vi "MainPr(Calculation)-40.vi"() -> ()   [LabVIEW 2013]
doc: "Main Program for Tracking\nThis VI Represents Front Panel and Control Buttons for Perform Tracking\nPlease, optimize the front panel for your own monitor resolution and needs"
uses:
  <vilib>/vision/Avi.llb/IMAQ AVI2 Refnum.ctl
  <vilib>/vision/NI_Vision_Development_Module.lvlib
panel:
  out "error out":errorcluster
  in  "STOP Program":bool
  in  "Front Panel":T1(tab)
  in  "FrameCtl":u32 max=499
  out "1st Movie (Comparison)":T2(plugin-control)
  out "1st Movie":T2(plugin-control)
  in  "Gamma":sgl format="%.2f"
  in  "Operator G Correction":T3(ring)
  in  "Parameter LoG":sgl format="%.2f"
  in  "Operator LoG":T3(ring)
  in  "1/2 Channels":bool
  in  "Sigma":dbl min=0.1
  in  "FrameCtl2":u32 max=499
  in  "Gray or Binarized?":bool
  out "1st Movie Original":T2(plugin-control)
  out "1st Movie Processed":T2(plugin-control)
  in  "Index for thresholding":i8 min=-9
  in  "Keep Nega-\ntive Values?":bool
  out "Detection Progress":u8(slide) scale=0.0..100.0
  in  "# of Frame":u32 max=499
  in  "Save pics (ex)":bool
  in  "Find ALL objects":bool
  out "Results on 1st Movie":T2(plugin-control)
  out "1st Filtering":T2(plugin-control)
  in  "Try my filters!":bool
  in  "# Erosion":i32=2
  in  "Connectivity":bool=TRUE
  in  "Min  Diam":dbl
  in  "Max  Diam":dbl min=12.0
  in  "Filter Tracks":bool
  out "Tracking progress":u8(slide) scale=0.0..100.0
  in  "Save pictures":bool
  in  "Save movies":bool
  in  "Frame":u32 max=499
  in  "Delete Tracs":bool
  out "1st Filtered":T2(plugin-control)
  in  "dR max":dbl min=1.0
  out "1st Filtering (NN)":T2(plugin-control)
  in  "dR min":dbl min=0.0 max=10.0
  out "Raw #":i32
  out "Saved #":i32
  in  "Tracking Procedure":bool
  in  "Min TRK L":i32 min=2 max=498 step=1
  in  "Closing gaps":i32 min=1 max=498 step=1
  in  "% linearity":i32 min=1 max=100 step=1
  in  "Max angle":dbl min=0.0 max=89.0 step=1.0
  in  "FPS":u32
  in  "FPS Gr":u32
  in  "Save videos \nbelow as *avi":bool
  in  "Save pics below":bool
  in  "Testing Frame":u32 max=17
  out "After Resolving Correspondence Problem":T2(plugin-control)
  out "Connected and Grouped Tracks":T2(plugin-control)
  in  "Tracks group":i32 min=0 max=394
  in  "Save Tracks in Columns (x,y,dx,dy)":bool
  in  "Save Duration of Tracks":bool
  in  "Save Mean Velocities":bool
  out "Duration of Tracks":T4(graph)
  out "Mean Instant Velocities for Each Track":T4(graph)
  in  "Show Distributions":bool
  out "All Path Vels":T4(graph)
  out "All Instant Vels":T4(graph)
  out "mean Instant Vel":dbl format="%#_1f"
  out "StD Instant":dbl format="%#_1g"
  out "mean Path Vel":dbl format="%.1f"
  out "StD Path":dbl format="%.1f"
  in  "Bins":i32=10
  in  "Save All Instant Vels":bool
  in  "Save Path Velocities":bool
  # "Two channels"
  # "*Planning develop-\nment switcher (old)"
  # "One channel"
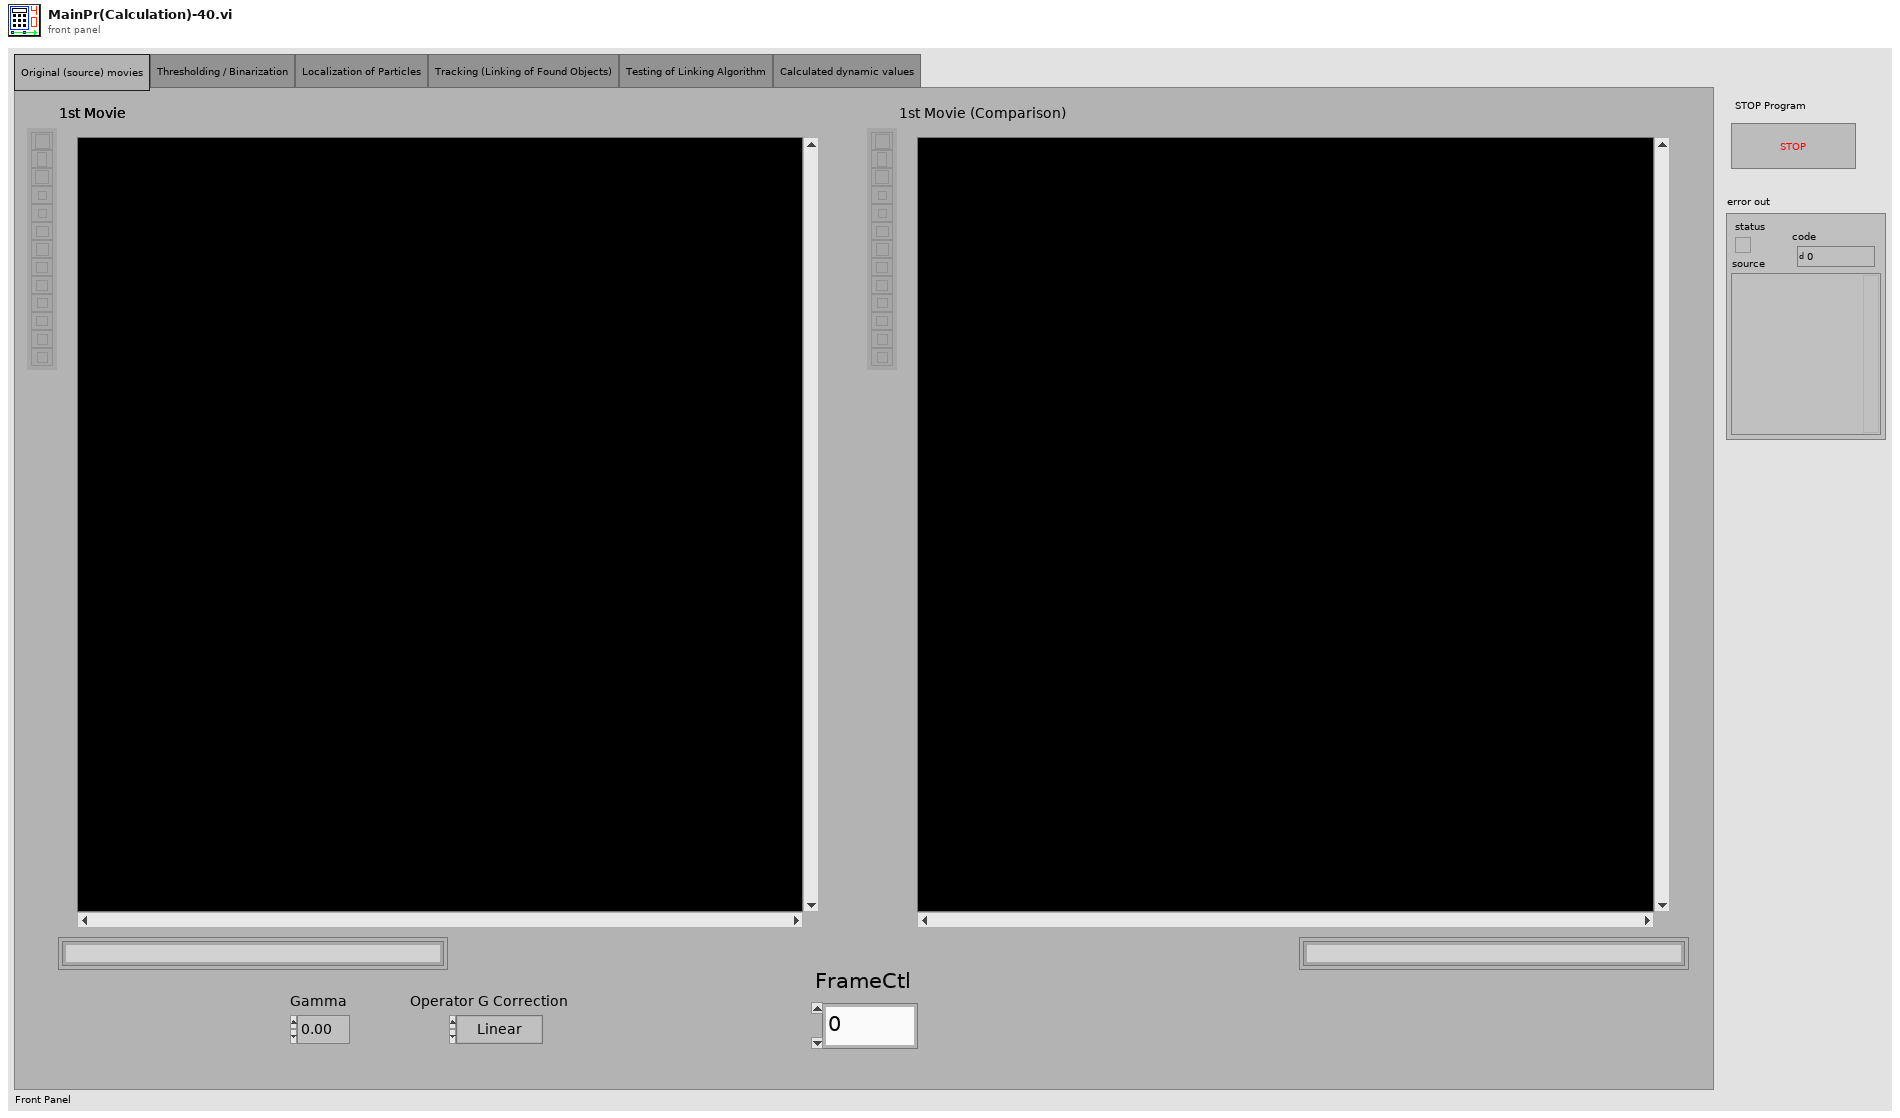
[diagram p1: front panel]
types:
  T1 = enum32{"Original (source) movies", "Thresholding / Binarization", "Localization of Particles", "Tracking (Linking of Found Objects)", "Testing of Linking Algorithm", "Calculated dynamic values"}
  T2 = typedef "IMAQ Image.ctl" = refnum<image>
  T3 = enum32{"Linear", "Log", "Exp", "Square", "Square root", "Power X", "Power 1/X"}
  T4 = cluster{"X Values":dbl[], "Histogram: h(x)":i32[]}
  T5 = typedef "IMAQ AVI2 Refnum.ctl" = refnum<k20>
  T6 = typedef "Image Type" = u32
  T7 = typedef "Particle Parameters" = i32
  T8 = cluster{"[IN] AVI Refnum":T5, "[IN] Image Type":T6, "[IN] Particle Filter Setups":cluster{"Erosion":i32, "Connectivity ":bool, "Type of particle filter":cluster{"Measurement Parameter":T7, "Min  Diam":dbl, "Max  Diam":dbl, "Range":bool, "Range":bool}[]}, "[IN] # Channel":u8, "[IN] Keep Nega-\ntive Values?":bool, "[IN] Image Filtering Settings":cluster{"Gamma Origin":sgl, "Operator Origin":enum32{"Linear", "Log", "Exp", "Square", "Square root", "Power X", "Power 1/X"}, "Gamma LoG":sgl, "Operator LoG":enum32{"Linear", "Log", "Exp", "Square", "Square root", "Power X", "Power 1/X"}, "Sigma":dbl, "Thresholding Index":i8}, "[IN] Binarization Settings":cluster{"MinBin2":sgl, "MaxBin2":sgl}[]}
  T9 = enum8{"Enabled", "Disabled", "Disabled and Grayed Out"}
  T10 = cluster{"dR min ":dbl, "dR max ":dbl, "Closing gaps":i32, "Min TRK L":i32, "% linearity":i32, "Max angle":dbl, "Tracking progress":refnum<vi>}
  T11 = cluster{"X,Y":dbl[][], "Areas particles":dbl[][], "Particle Fil Setups":cluster{"Erosion":i32, "Connectivity ":bool, "Type of particle filter":cluster{"Measurement Parameter":T7, "Min  Diam":dbl, "Max  Diam":dbl, "Range":bool, "Range":bool}[]}, "Tracks, Coordinates":cluster{"(X,Y) Unmoved":dbl[][], "(X,Y,dX,dY) Dur 1 Frame":dbl[][], "(X,Y,dX,dY) W/t Problems":dbl[][], "(X,Y,dX,dY) NN filtered":dbl[][], "(X,Y,dX,dY) TH filtered":dbl[][], "Tracks":cluster{"Tracks":dbl[], "Start Pos":i32}[], "Tracks w/t Problems":cluster{"Tracks":dbl[], "Start Pos":i32}[]}}
  T12 = cluster{"Gamma Origin":sgl, "Operator Origin":enum32{"Linear", "Log", "Exp", "Square", "Square root", "Power X", "Power 1/X"}, "Gamma LoG":sgl, "Operator LoG":enum32{"Linear", "Log", "Exp", "Square", "Square root", "Power X", "Power 1/X"}, "Sigma":dbl, "Thresholding Index":i8}
  T13 = cluster{"Before Grouped Tracks":cluster{"Tracks":dbl[][], "Start Pos":i32[], "Dot Statuses":i16[][]}[], "After Grouped Tracks":cluster{"Tracks":dbl[][], "Start Pos":i32[], "Dot Statuses":i16[][]}[], "Current\nGroup":i32}
  T14 = cluster{"Instant Velocities (All)":dbl[], "Path Velocities (All) ":dbl[], "Tracks in columns":dbl[][], "Mean Instant Velo\ncities for Tracks":dbl[], "MSD":dbl[], "Track duration in frames":u16[], "Track length in pixels":dbl[]}
  T15 = cluster{"Starting Value":sgl, "Incremental Value":sgl, "Histogram":u32[]}
  T16 = cluster{"Erosion":i32, "Connectivity ":bool, "Type of particle filter":cluster{"Measurement Parameter":T7, "Min  Diam":dbl, "Max  Diam":dbl, "Range":bool, "Range":bool}[]}
  T17 = cluster{"Measurement Parameter":T7, "Min  Diam":dbl, "Max  Diam":dbl, "Range":bool, "Range":bool}[]
  T18 = cluster{"Tracks W/T Problems":dbl[], "Start Pos":i32}[]
  T19 = cluster{"All Instant Vel-s":cluster{"X Values":dbl[], "Histogram: h(x)":i32[]}, "mean":dbl, "standard deviation":dbl, "All Path Vel-s":cluster{"X Values":dbl[], "Histogram: h(x)":i32[]}, "mean":dbl, "standard deviation":dbl, "Mean Instan Vel-s":cluster{"X Values":dbl[], "Histogram: h(x)":i32[]}, "mean":dbl, "standard deviation":dbl, "Duration of tracks":cluster{"X Values":dbl[], "Histogram: h(x)":i32[]}, "mean":dbl, "standard deviation":dbl}
  T20 = cluster{"(X,Y) Unmoved":dbl[][], "(X,Y,dX,dY) Dur 1 Frame":dbl[][], "(X,Y,dX,dY) W/t Problems":dbl[][], "(X,Y,dX,dY) NN filtered":dbl[][], "(X,Y,dX,dY) TH filtered":dbl[][], "Tracks":cluster{"Tracks":dbl[], "Start Pos":i32}[], "Tracks w/t Problems":cluster{"Tracks":dbl[], "Start Pos":i32}[]}
  T21 = cluster{"Tracks":dbl[][], "Start Pos":i32[], "Dot Statuses":i16[][]}[]
  T22 = cluster{"[IN] Grouped Tracks":cluster{"Tracks":dbl[][], "Start Pos":i32[], "Dot Statuses":i16[][]}[], "[IN] Tracks group":i32, "[IN] Testing Frame ":u32}
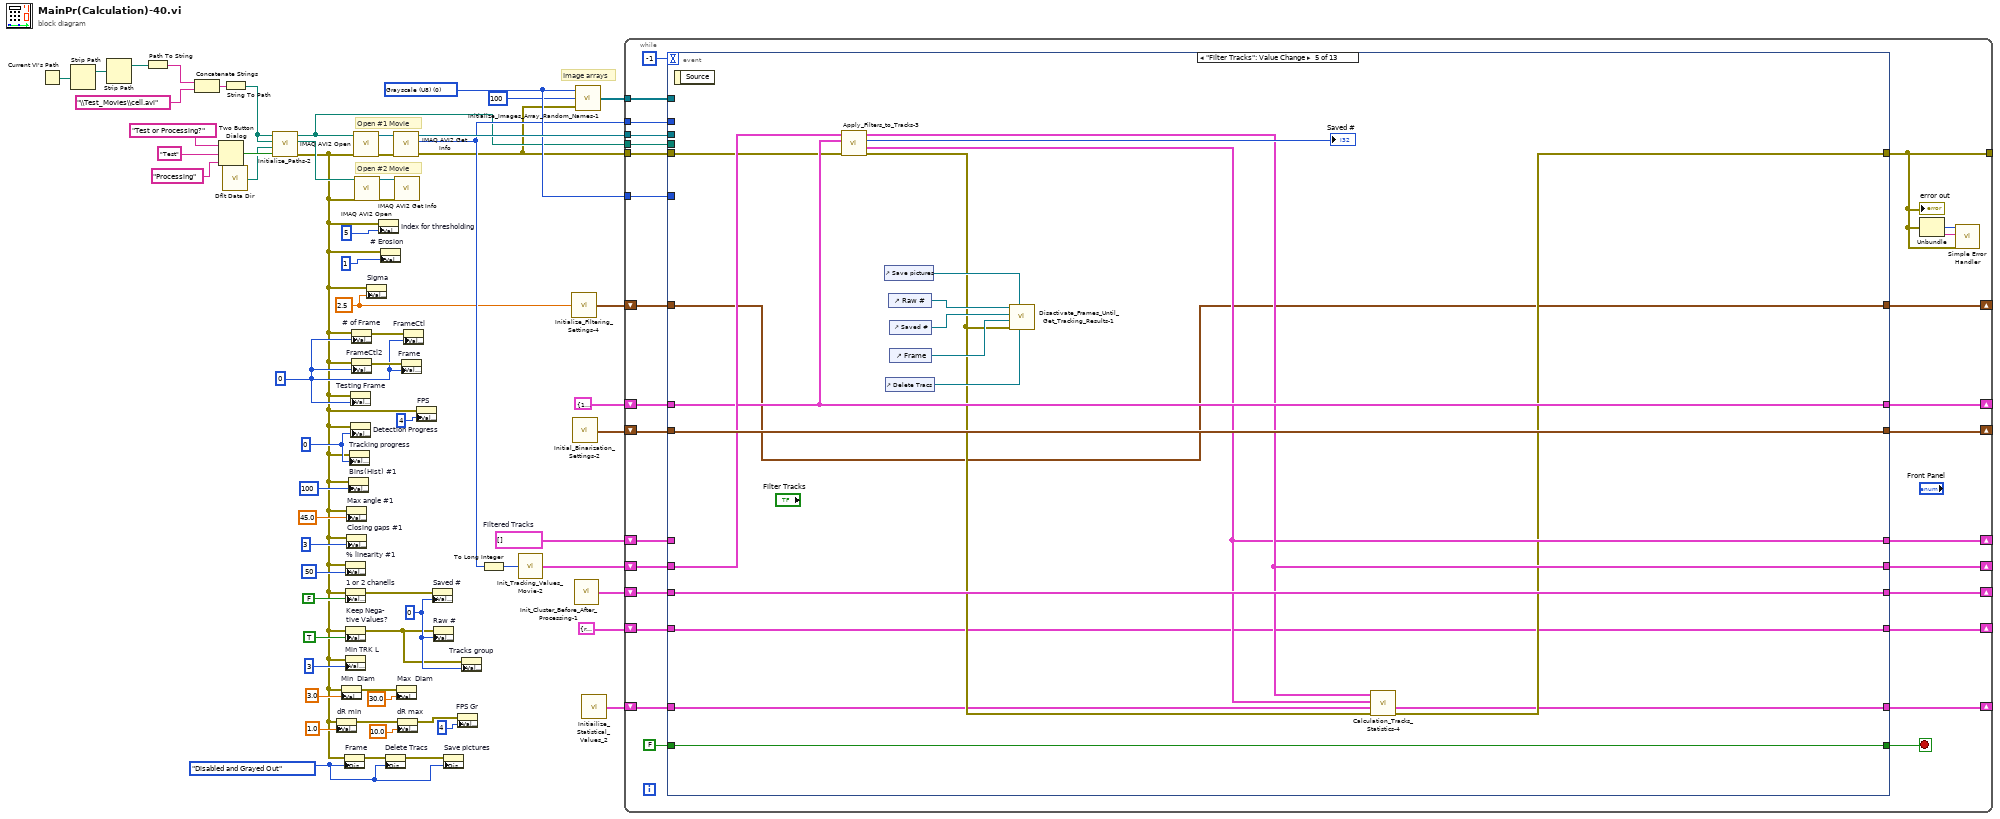
[diagram p0: block diagram]
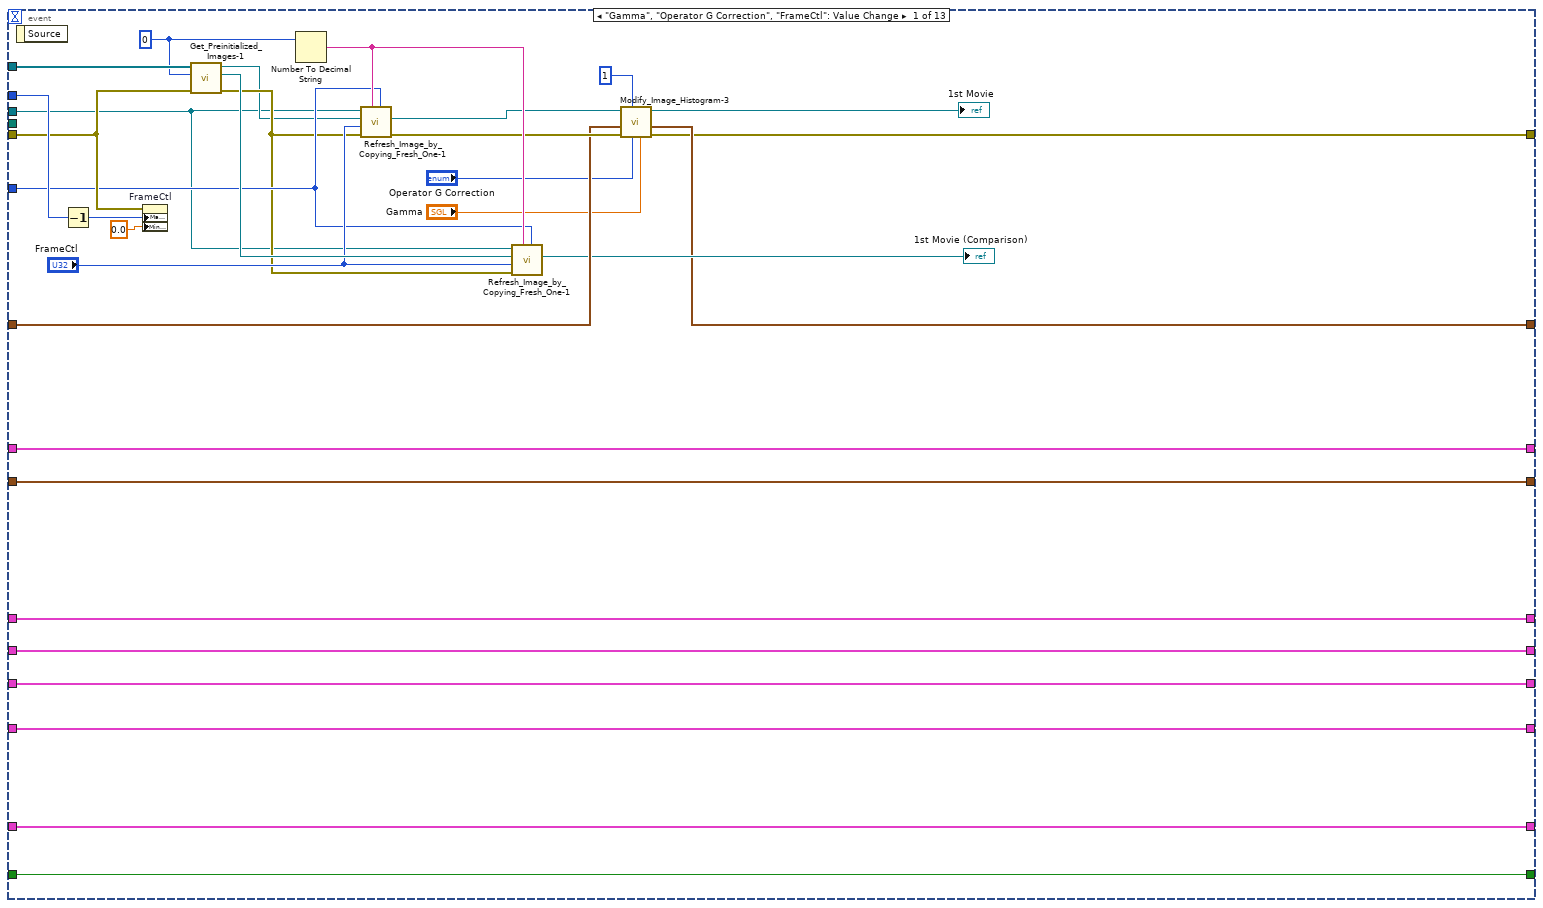
[diagram p2: hidden frame]
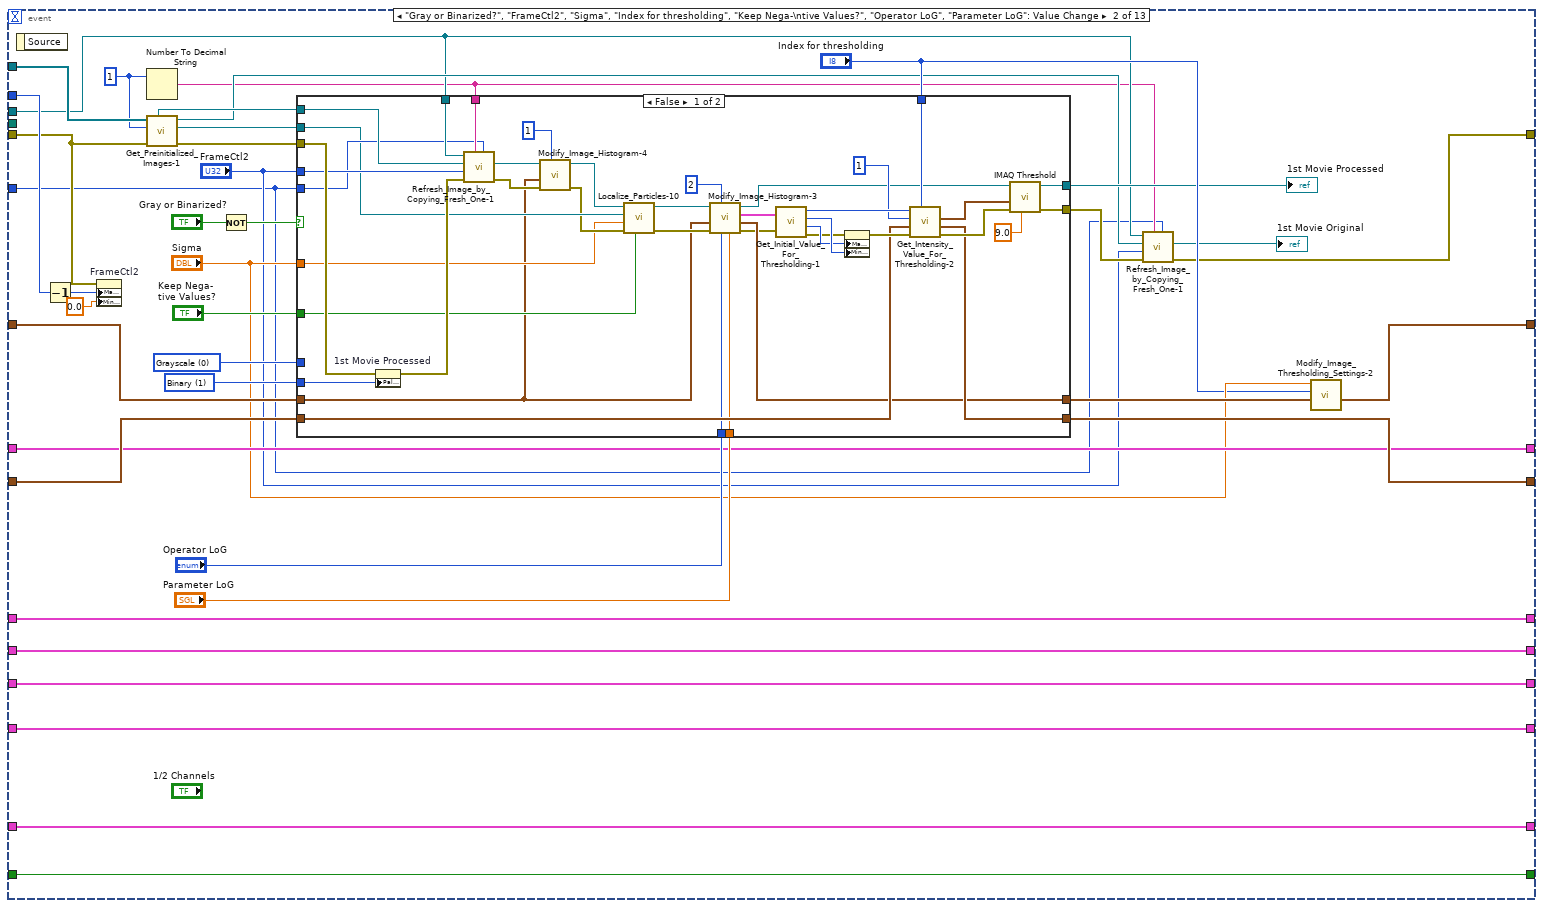
[diagram p3: hidden frame]
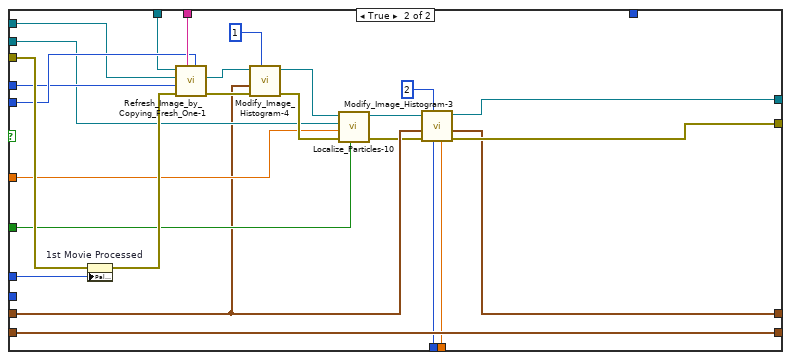
[diagram p4: hidden frame]
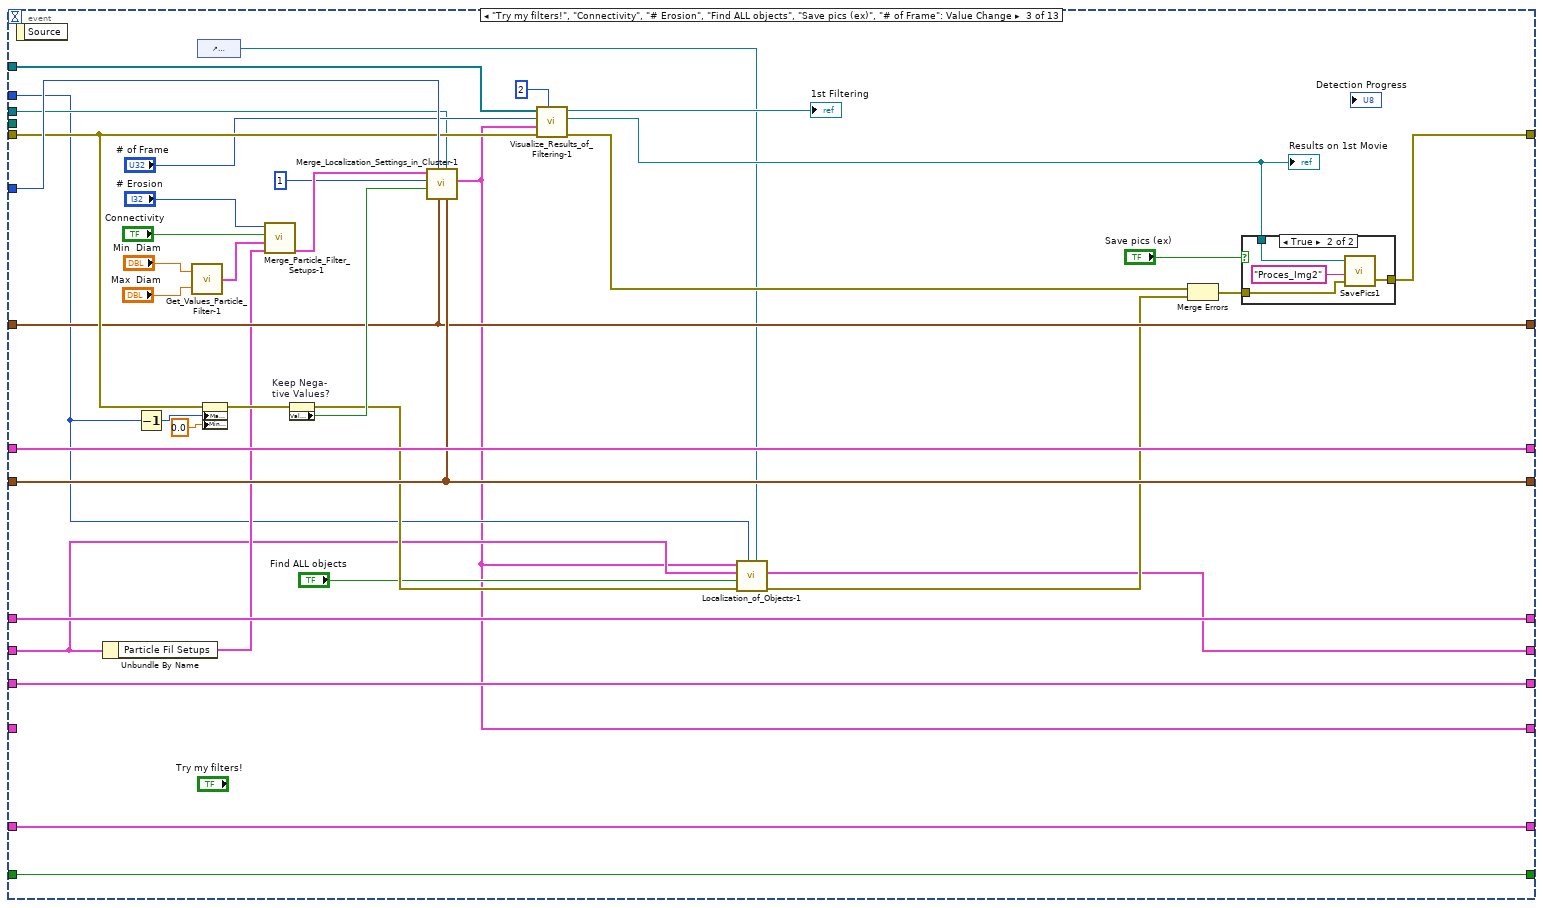
[diagram p5: hidden frame]
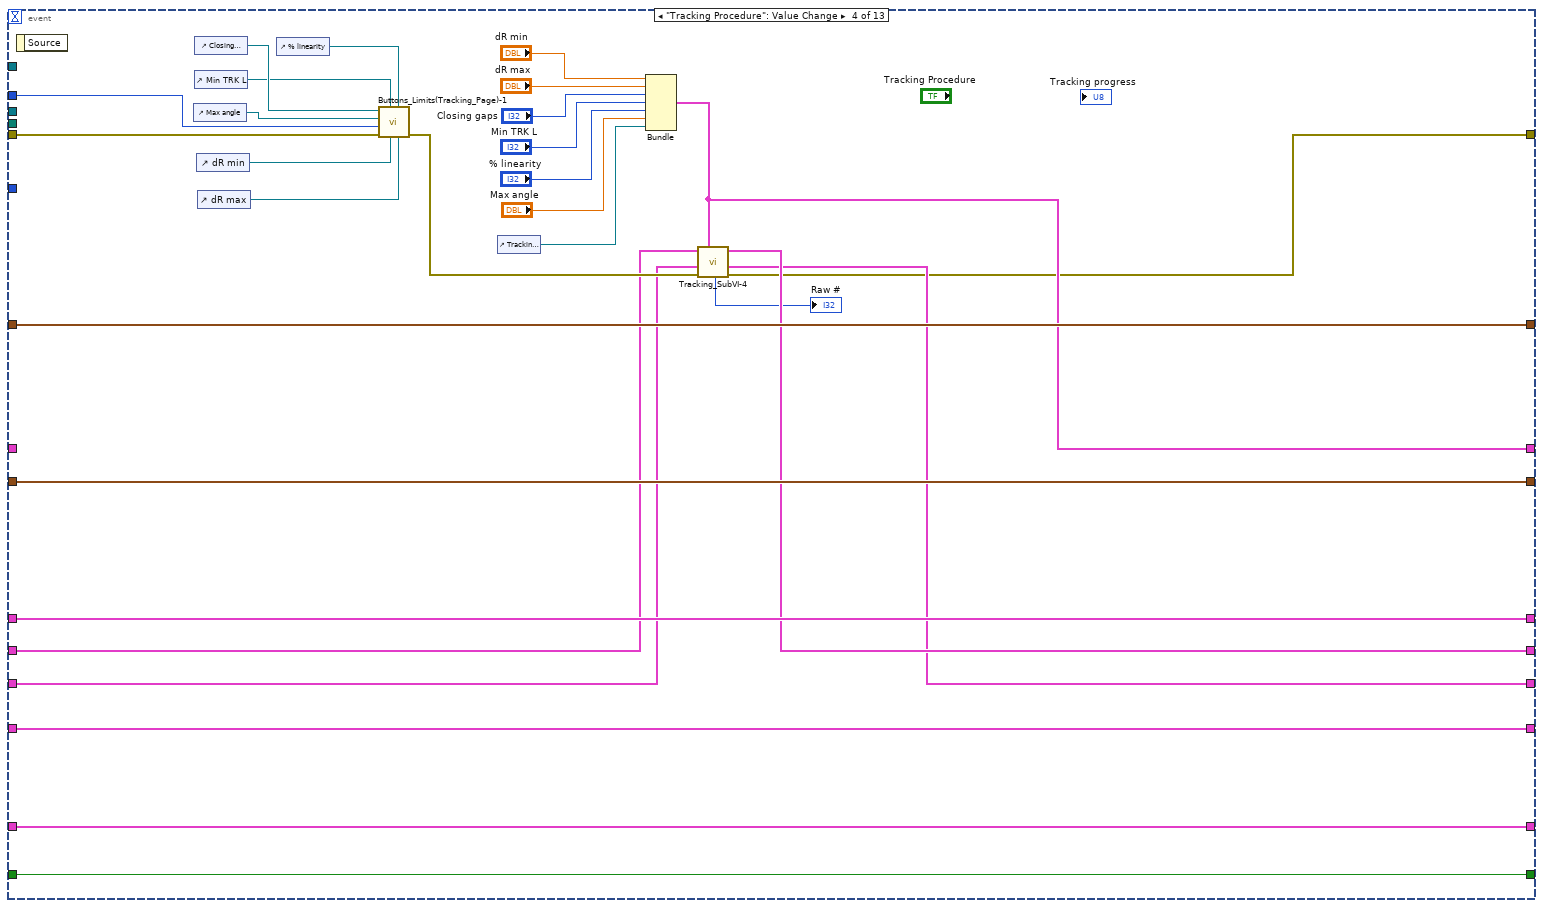
[diagram p7: hidden frame]
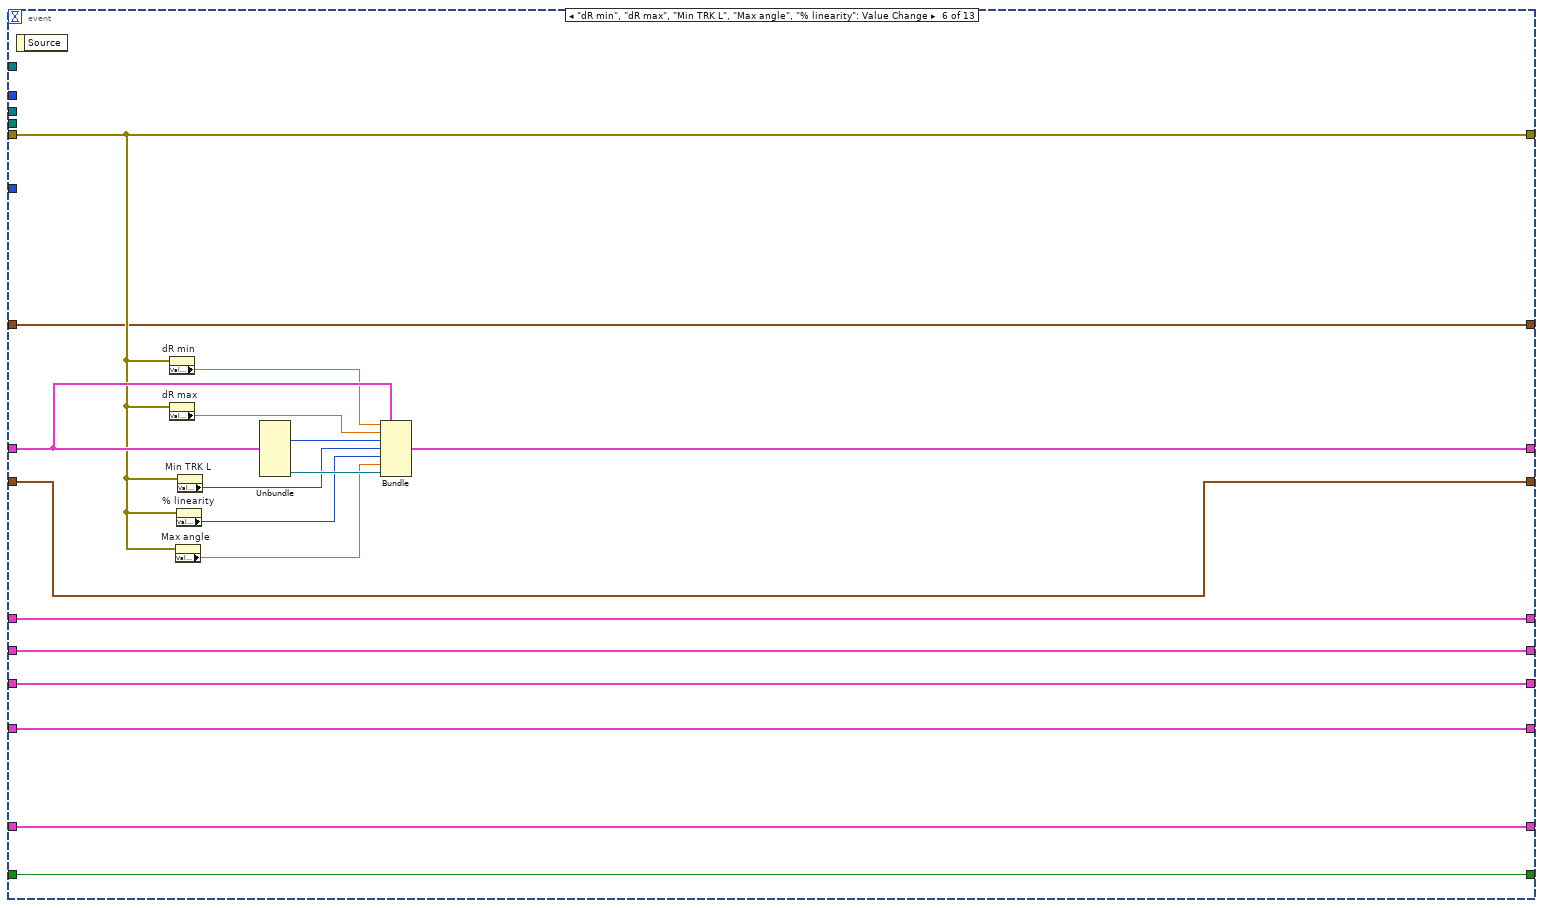
[diagram p8: hidden frame]
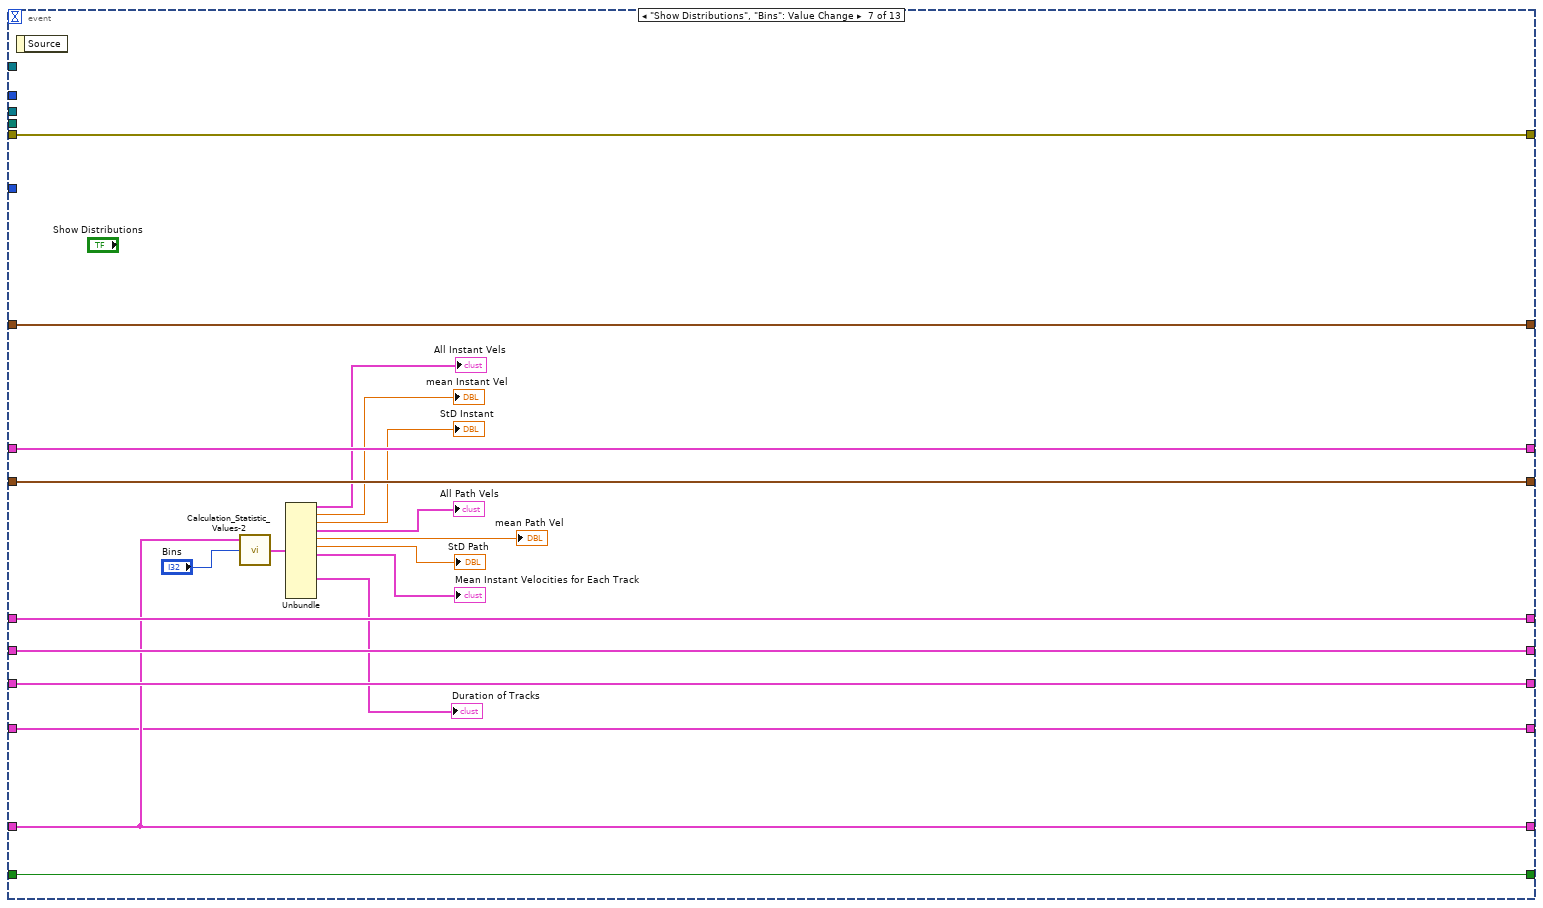
[diagram p9: hidden frame]
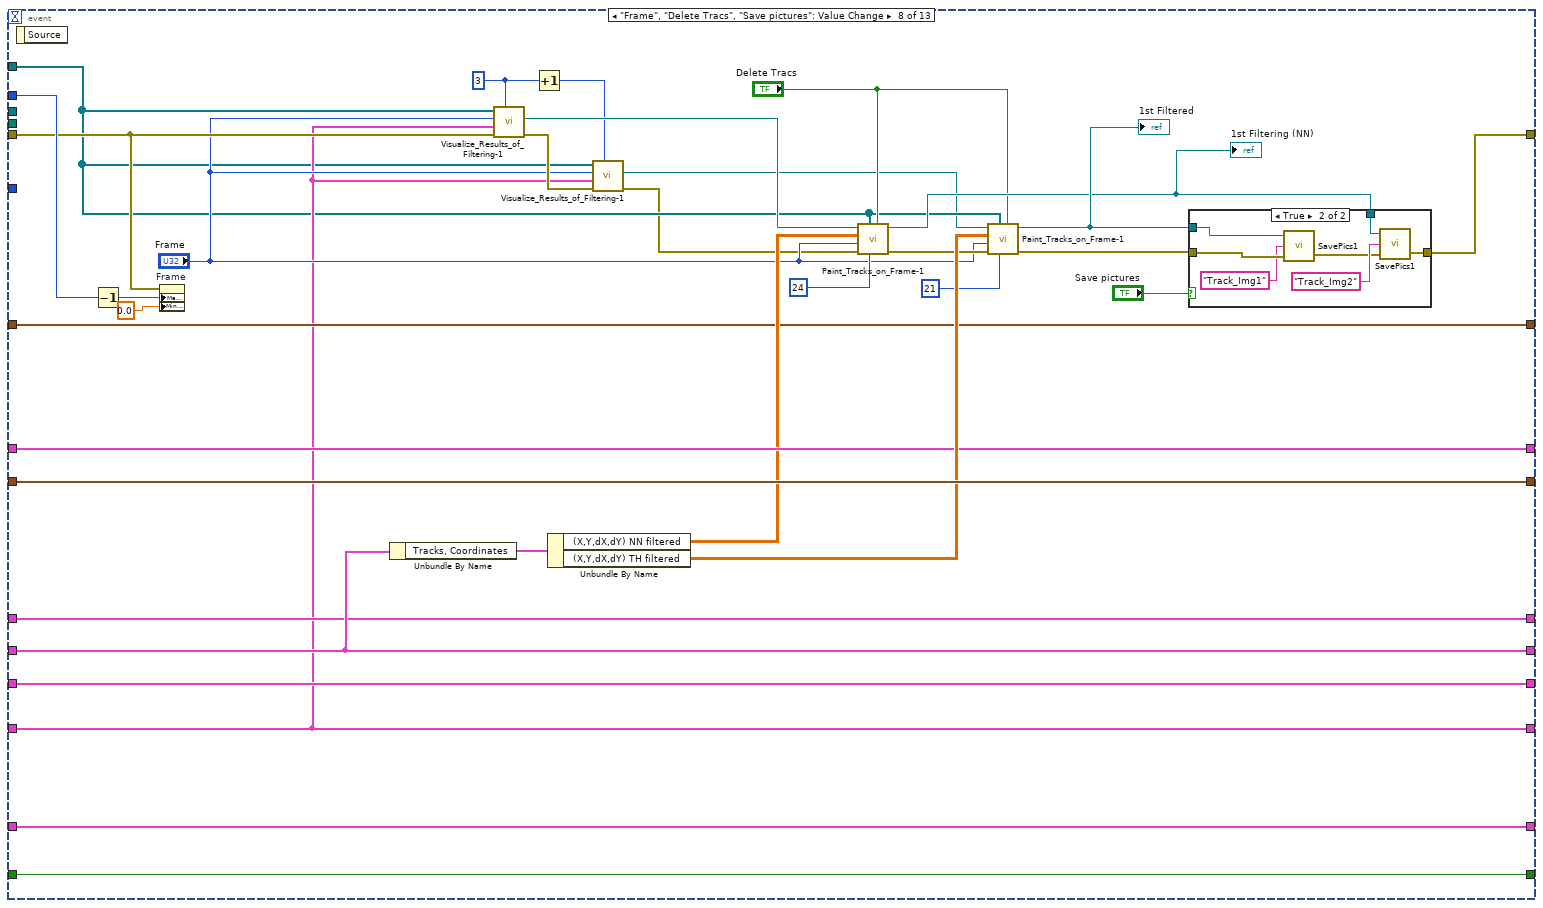
[diagram p10: hidden frame]
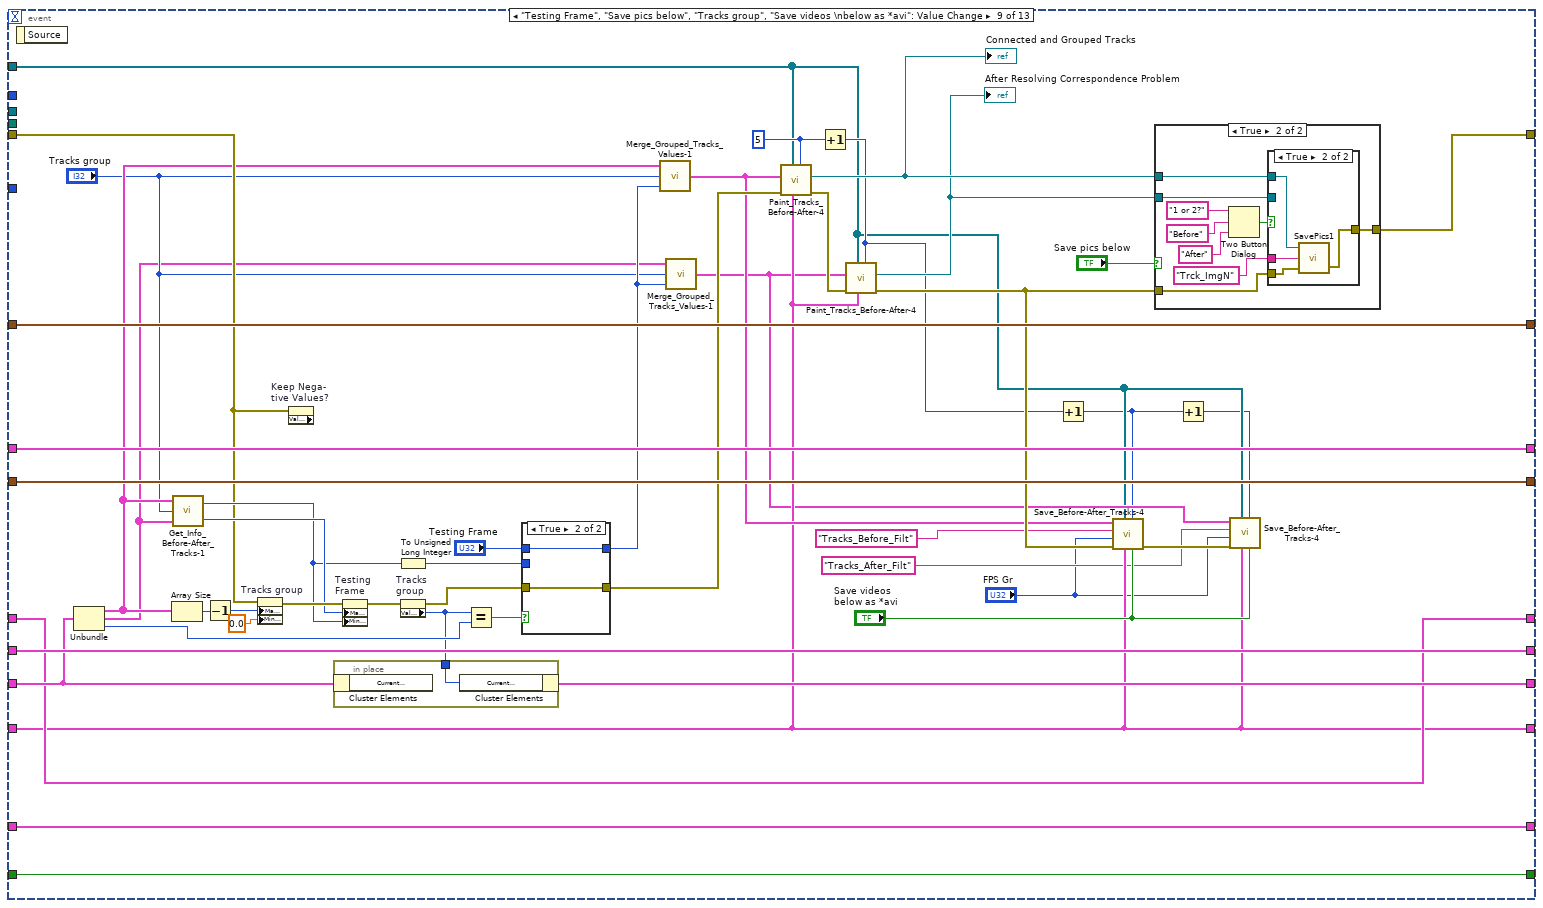
[diagram p12: hidden frame]
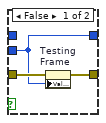
[diagram p13: hidden frame]
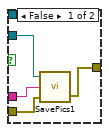
[diagram p15: hidden frame]
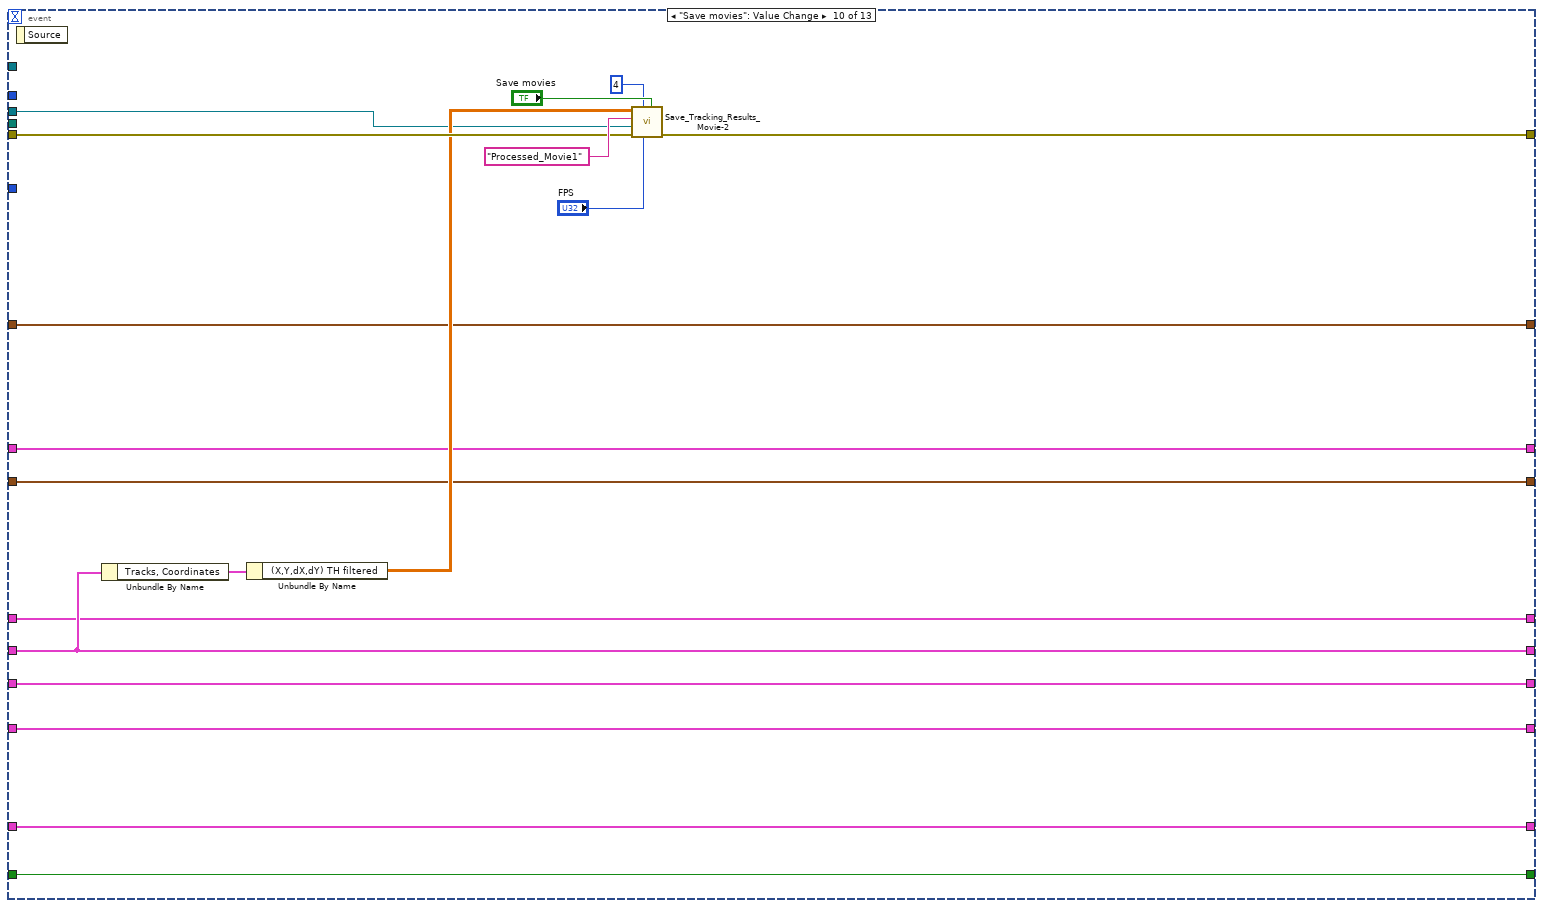
[diagram p16: hidden frame]
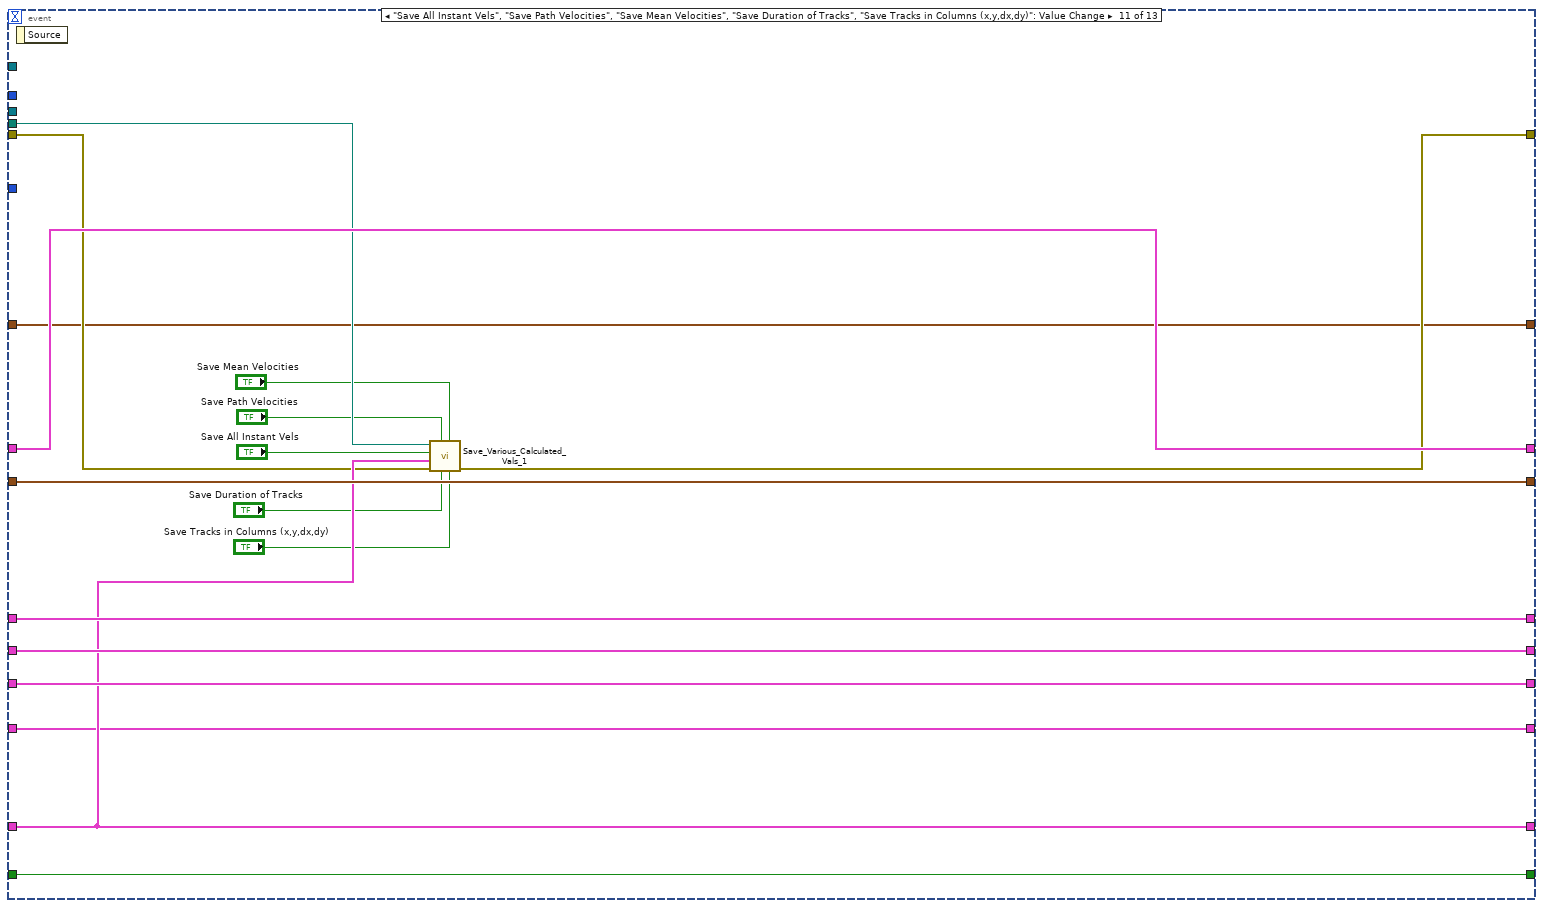
[diagram p17: hidden frame]
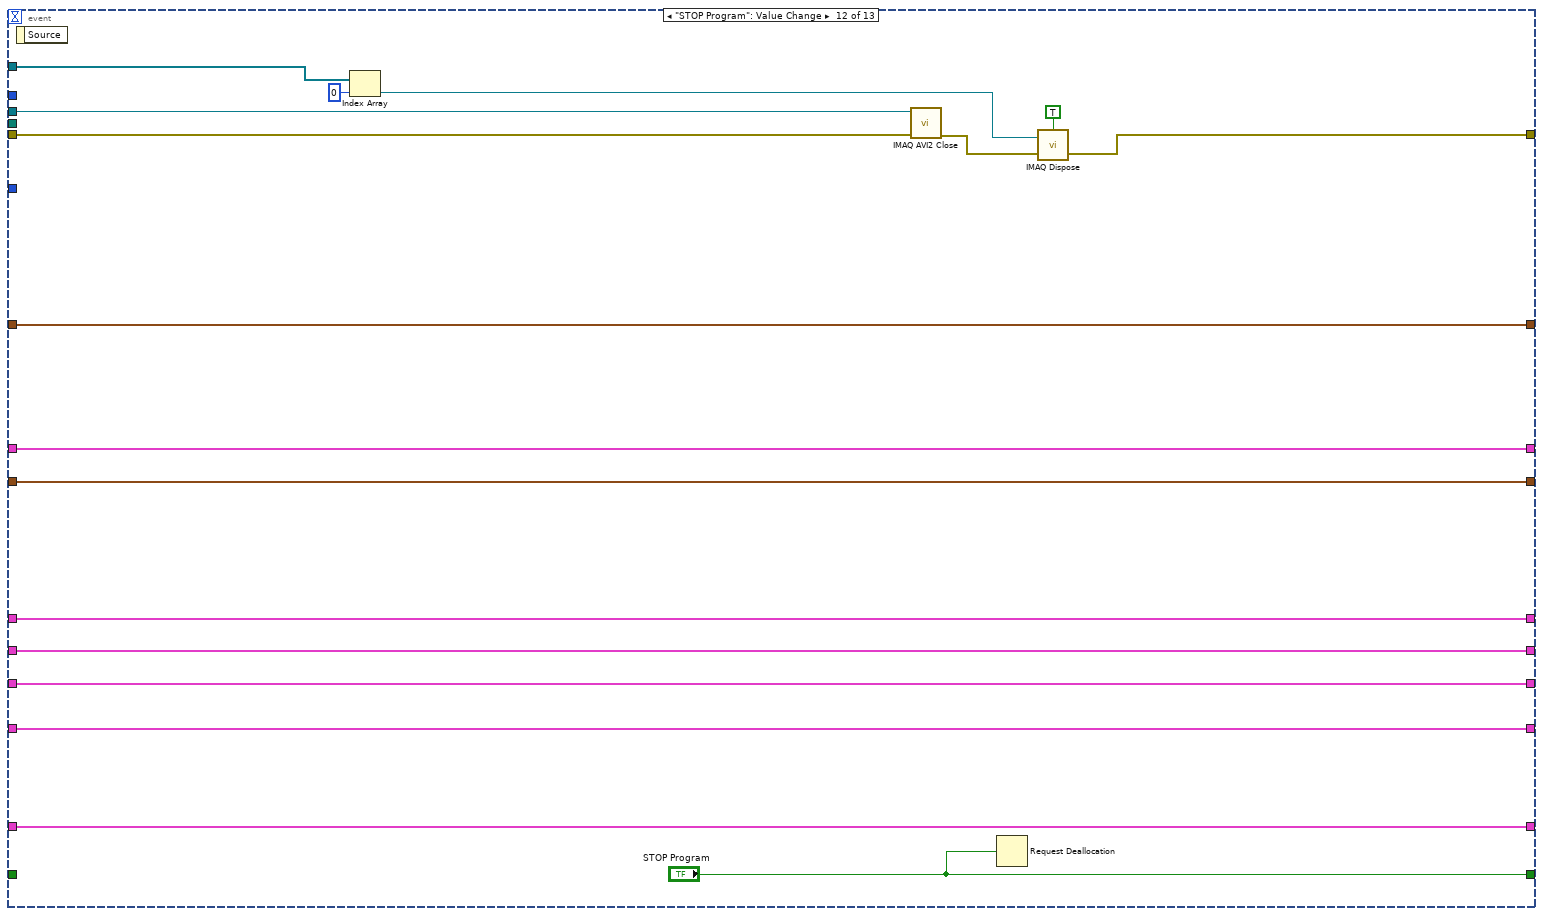
[diagram p18: hidden frame]
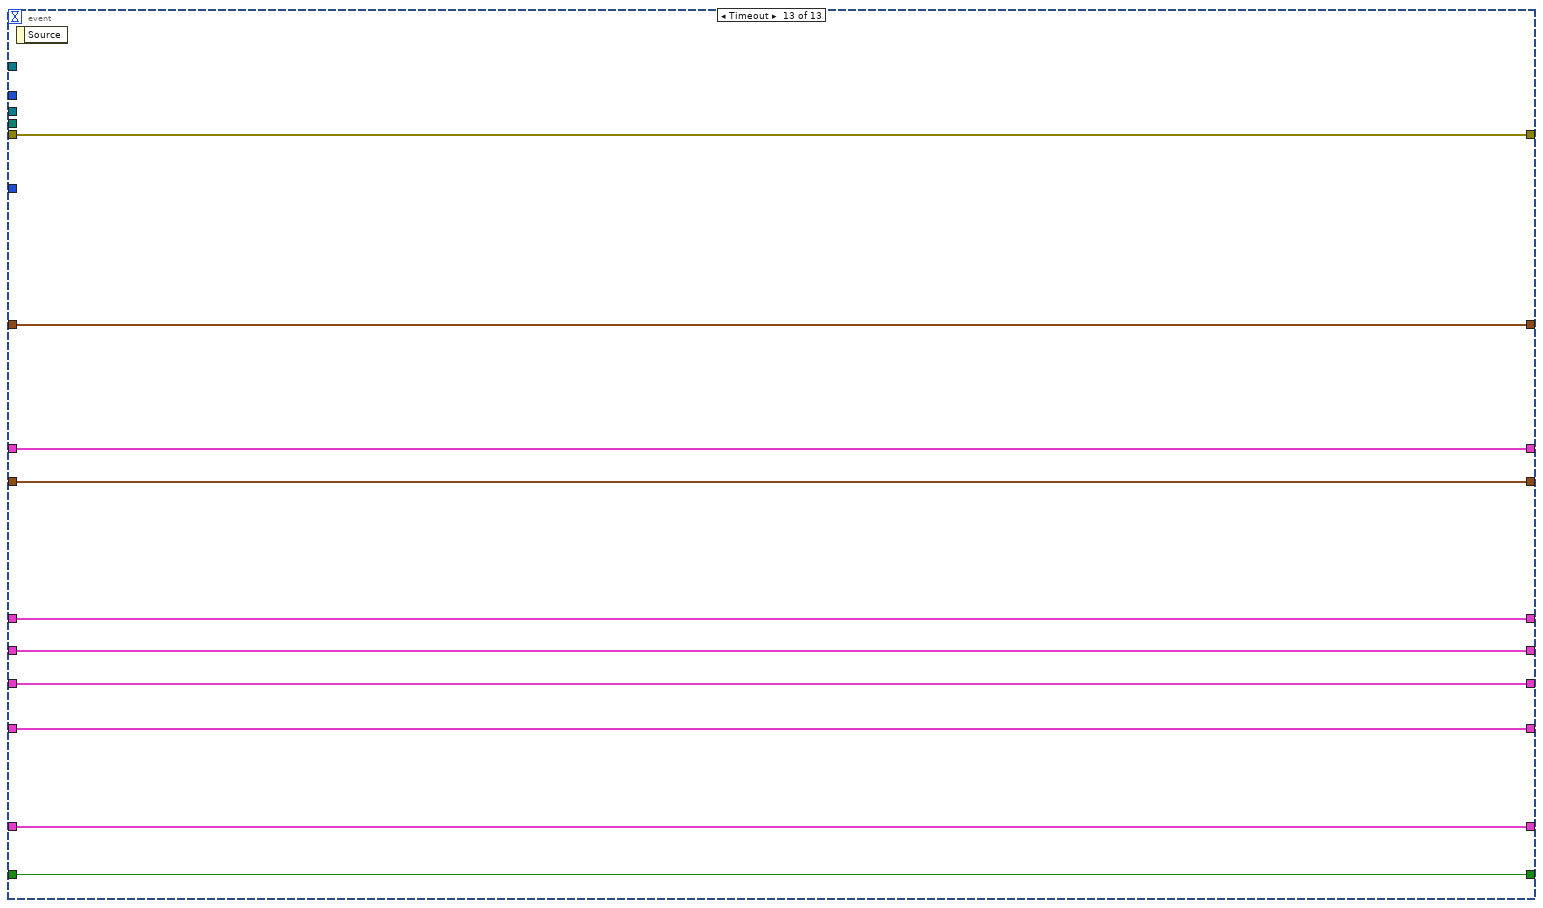
[diagram p19: hidden frame]
diagram:
  w10 = 0 ("Saved #")
  w14 = cluster{"Tracks":dbl[], "Start Pos":i32}[] []  # Filtered Tracks
  w15 = T9."Disabled and Grayed Out" ("Disabled")
  w11 = u32 0 ("Testing Frame")
  w33 = u8 0 ("Progress")
  w5 = 2.5 ("Sigma")
  w41 = T6 0 items=["Grayscale (U8)", "Grayscale (I16)", "Grayscale (SGL)", "Complex (CSG)", "RGB (U32)", "HSL (U32)", "RGB (U64)", "Grayscale (U16)"] ("Image Type")
  # "Image arrays"
  # "Open #2 Movie"
  # "Open #1 Movie"
  n1 = Current VI's Path() -> (path=w26:path)
  n2 = Strip Path(path=w26) -> (stripped path=w22:path)  [unwired: 1 out]
  n3 = Strip Path(path=w22) -> (stripped path=w21:path)  [unwired: 1 out]
  n4 = Path To String(path=w21) -> (string=w31:string)
  n5 = Concatenate Strings(w31, "\\Test_Movies\\cell.avi" ("string")) -> (w28:string)
  n6 = Two Button Dialog(message="Test or Processing?", 1:"Processing" ("F button name (\"Cancel\")"), 2:"Test" ("T button name (\"OK\")")) -> (T button?=w37:bool)
  n7 = call <vilib>:"Dflt Data Dir.vi"() -> ("App:Default Data Directory"=w29:path)
  n8 = String To Path(string=w28) -> (path=w27:path)
  n9 = call "Initialize_Paths-2.vi"("Test or Processing?"=w37, "start path"=w29, "AVI File Path #2"=w27, "AVI File Path #1"=w27) -> ("ERROR OUT"=w8:errorcluster, "AVI File Path #2 OUT"=w36:path, "AVI File Path #1 OUT"=w25:path)  [unwired: 1 out]
  n10 = property on="dR min" class="DigNum (strict)"(error in=w8, "Value"=1.0 ("dR min")) -> (error out=w45:errorcluster)  [unwired: 1 in, 1 out]
  n11 = property on="Min  Diam" class="DigNum (strict)"(error in=w8, "Value"=3.0 ("Min  Diam")) -> (error out=w48:errorcluster)  [unwired: 1 in, 1 out]
  n12 = property on="Frame" class="DigNum (strict)"(error in=w8, "DisabledEnum"=w15) -> (error out=w17:errorcluster)  [unwired: 1 in, 1 out]
  n13 = property on="Min TRK L" class="DigNum (strict)"(error in=w8, "Value"=3 ("Min TRK L")) -> ()  [unwired: 1 in, 2 out]
  n14 = property on="% linearity #1" class="DigNum (strict)"(error in=w8, "Value"=50 ("% linearity")) -> ()  [unwired: 1 in, 2 out]
  n15 = property on="1 or 2 chanells" class="Bool (strict)"(error in=w8, "Value"=FALSE) -> (error out=w13:errorcluster)  [unwired: 1 in, 1 out]
  n16 = property on="Keep Nega-\ntive Values?" class="Bool (strict)"(error in=w8, "Value"=TRUE ("Keep Nega-\ntive Values?")) -> (error out=w9:errorcluster)  [unwired: 1 in, 1 out]
  n17 = property on="Max angle #1" class="DigNum (strict)"(error in=w8, "Value"=45.0 ("Max angle")) -> ()  [unwired: 1 in, 2 out]
  n18 = property on="Closing gaps #1" class="DigNum (strict)"(error in=w8, "Value"=3 ("Closing gaps")) -> ()  [unwired: 1 in, 2 out]
  n19 = property on="Bins(Hist) #1" class="DigNum (strict)"(error in=w8, "Value"=100 ("Intervals")) -> ()  [unwired: 1 in, 2 out]
  n20 = property on="Tracking progress" class="Slide (strict)"(error in=w8, "Value"=w33) -> ()  [unwired: 1 in, 2 out]
  n21 = property on="Testing Frame" class="DigNum (strict)"(error in=w8, "Value"=w11) -> ()  [unwired: 1 in, 2 out]
  n22 = property on="Detection Progress" class="Slide (strict)"(error in=w8, "Value"=w33) -> ()  [unwired: 1 in, 2 out]
  n23 = property on="# of Frame" class="DigNum (strict)"(error in=w8, "Value"=w11) -> (error out=w24:errorcluster)  [unwired: 1 in, 1 out]
  n24 = property on="FrameCtl2" class="DigNum (strict)"(error in=w8, "Value"=w11) -> (error out=w23:errorcluster)  [unwired: 1 in, 1 out]
  n25 = call "IMAQ AVI2 Open"("error in (no error)"=w8, "AVI File Path"=w25) -> ("error out"=w62:errorcluster, "AVI Refnum"=w63:T5)  [unwired: 8 in]
  n26 = call "IMAQ AVI2 Open"("error in (no error)"=w8, "AVI File Path"=w36) -> ("error out"=w61:errorcluster, "AVI Refnum"=w60:T5)  [unwired: 8 in]
  n27 = property on="Sigma" class="DigNum (strict)"(error in=w8, "Value"=w5) -> ()  [unwired: 1 in, 2 out]
  n28 = property on="Index for thresholding" class="DigNum (strict)"(error in=w8, "Value"=i8 5 ("Index for \nthresholding")) -> ()  [unwired: 1 in, 2 out]
  n29 = property on="# Erosion" class="DigNum (strict)"(error in=w8, "Value"=1 ("# Erosion")) -> ()  [unwired: 1 in, 2 out]
  n30 = property on="Delete Tracs" class="Bool"(error in=w17, "DisabledEnum"=w15) -> (error out=w16:errorcluster)  [unwired: 1 in, 1 out]
  n31 = call "IMAQ AVI2 Get Info"("error in (no error)"=w62, "AVI Refnum"=w63) -> ("error out"=w12:errorcluster, "Number of Frames"=w40:u32, "AVI Refnum (duplicate)"=w59:T5)  [unwired: 5 in, 2 out]
  n32 = call "IMAQ AVI2 Get Info"("error in (no error)"=w61, "AVI Refnum"=w60) -> ()  [unwired: 5 in, 5 out]
  n33 = property on="Max  Diam" class="DigNum (strict)"(error in=w48, "Value"=30.0 ("Max  Diam")) -> ()  [unwired: 1 in, 2 out]
  n34 = property on="dR max" class="DigNum (strict)"(error in=w45, "Value"=10.0 ("dR max")) -> (error out=w1:errorcluster)  [unwired: 1 in, 1 out]
  n35 = property on="Frame" class="DigNum (strict)"(error in=w23, "Value"=w11) -> ()  [unwired: 1 in, 2 out]
  n36 = property on="FrameCtl" class="DigNum (strict)"(error in=w24, "Value"=w11) -> ()  [unwired: 1 in, 2 out]
  n37 = property on="FPS" class="DigNum (strict)"(error in=w8, "Value"=u32 4 ("FPS")) -> ()  [unwired: 1 in, 2 out]
  n38 = property on="Saved #" class="DigNum (strict)"(error in=w13, "Value"=w10) -> ()  [unwired: 1 in, 2 out]
  n39 = property on="Raw #" class="DigNum (strict)"(error in=w9, "Value"=w10) -> ()  [unwired: 1 in, 2 out]
  n40 = property on="Save pictures" class="Bool"(error in=w16, "DisabledEnum"=w15) -> ()  [unwired: 1 in, 2 out]
  n41 = property on="FPS Gr" class="DigNum (strict)"(error in=w1, "Value"=u32 4 ("FPS Gr")) -> ()  [unwired: 1 in, 2 out]
  n42 = property on="Tracks group" class="DigNum (strict)"(error in=w9, "Value"=w10) -> ()  [unwired: 1 in, 2 out]
  n43 = To Long Integer(number=w40) -> (32bit integer=w19:i32)
  n44 = call "Init_Tracking_Values_Movie-2.vi"("[IN] # Frames"=w19) -> ("[OUT] Movie Values\n(Empty Cluster)"=w18:T11)
  n45 = call "Initialize_Filtering_Settings-4.vi"("Sigma #1"=w5) -> ("[OUT] Image Filtering Settings"=w4:T12)
  n46 = call "Initial_Binarization_Settings-2.vi"() -> ("Binarization Settings"=w43:cluster{"MinBin2":sgl, "MaxBin2":sgl}[])
  n47 = call "Init_Cluster_Before_After_Processing-1.vi"() -> ("[OUT] Before-After"=w35:T13)
  n48 = call "Initialize_Images_Array_Random_Names-1.vi"("error IN"=w12, "# Pics"=100, "Image Type"=w41) -> ("Images Array"=w39:T2[])
  n49 = call "Initiailize_Statistical_Values_2.vi"() -> ("Statistics"=w6:T14)
  n50 = while {
    tunnel: w12 -> [w85]
    tunnel: w40 -> [w88]
    tunnel: [w80] -> _
    tunnel: w59 -> [w89]
    shift-right: [w83] -> _
    shift-left: w18 -> [w84]
    shift-right: [w81] -> _
    shift-left: w6 -> [w82]
    shift-right: [w78] -> _
    shift-left: w35 -> [w79]
    shift-right: [w76] -> _
    shift-left: w43 -> [w77]
    tunnel: w41 -> [w75]
    tunnel: w39 -> [w74]
    tunnel: w25 -> [w72]
    shift-right: [w71] -> _
    shift-left: T10 {"dR min "=1.0, "dR max "=10.0, "Closing gaps"=3, "Min TRK L"=3, "% linearity"=50, "Max angle"=46.0, "Tracking progress"=refnum} -> [w70]
    shift-right: [w68] -> _
    shift-left: w14 -> [w69]
    shift-right: [w66] -> _
    shift-left: w4 -> [w67]
    shift-right: [w64] -> _
    shift-left: T8 {"[IN] AVI Refnum"=refnum, "[IN] Image Type"=0, "[IN] Particle Filter Setups"={"Erosion"=0, "Connectivity "=FALSE, "Type of particle filter"=[]}, "[IN] # Channel"=0, "[IN] Keep Nega-\ntive Values?"=FALSE, "[IN] Image Filtering Settings"={"Gamma Origin"=0.0, "Operator Origin"=enum."Linear", "Gamma LoG"=0.0, "Operator LoG"=enum."Linear", "Sigma"=0.0, "Thresholding Index"=0}, "[IN] Binarization Settings"=[]} ("[OUT] Localization Settings") -> [w65]
    stop <- w91 stop-if-true
    n51 = event shown="[4] \"Filter Tracks\": Value Change" {
      selector: _ -> [_ _ _ _ _ _ _ _ _ _ _ _ _]
      dyn-events: _ -> [_ _ _ _ _ _ _ _ _ _ _ _ _]
      timeout: -1 -> [_ _ _ _ _ _ _ _ _ _ _ _ _]
      tunnel: [w105 w141 w256 w284 w315 w332 w354 w377 w429 w477 w502 "STOP Program" w527] -> w91
      tunnel: w89 -> [w106 w127 w238 _ _ _ _ _ _ w481 _ w516 _]
      tunnel: w85 -> [w115 w151 w244 w299 w310 w326 w358 w368 w422 w484 w496 w515 w532]
      tunnel: w88 -> [w116 w152 w233 w298 _ _ _ w383 _ _ _ _ _]
      tunnel: [w93 w130 w262 w273 w305 w326 w358 w390 w439 w478 w497 w511 w532] -> w80
      tunnel: w84 -> [w122 w156 w229 w277 w312 w335 w356 w389 w444 w487 w505 w522 w531]
      tunnel: [w122 w156 w231 w275 w308 w335 w356 w389 w444 w487 w505 w522 w531] -> w83
      tunnel: w82 -> [w119 w157 w264 w282 w304 w333 w351 w386 w446 w488 w498 w520 w530]
      tunnel: [w119 w157 w264 w282 w303 w333 w351 w386 w446 w488 w498 w520 w530] -> w81
      tunnel: w79 -> [w118 w155 w261 w278 w314 w334 w355 w384 w428 w486 w504 w519 w529]
      tunnel: [w118 w155 w261 w274 w314 w334 w355 w384 w426 w486 w504 w519 w529] -> w78
      tunnel: w77 -> [w117 w154 w247 w300 w313 w324 w357 w382 w430 w479 w503 w518 w528]
      tunnel: [w117 w153 w247 w300 w313 w324 w357 w382 w430 w479 w503 w518 w528] -> w76
      tunnel: w75 -> [w109 w125 w246 _ _ _ _ _ _ _ _ _ _]
      tunnel: w74 -> [w114 w150 w243 _ _ _ _ w361 w403 _ _ w517 _]
      tunnel: FALSE ("STOP Program") -> [w105 w141 w256 w284 w315 w332 w354 w377 w429 w477 w502 _ w527]
      tunnel: w72 -> [_ _ _ _ _ _ _ _ _ _ w495 _ _]
      tunnel: [w104 w140 w255 w276 w311 w323 w353 w376 w425 w476 w501 w510 w526] -> w71
      tunnel: w70 -> [w104 w140 w255 _ w311 w338 w353 w376 w425 w476 w501 w510 w526]
      tunnel: w69 -> [w103 w139 w254 w283 _ w336 w352 w375 w424 w475 w500 w509 w525]
      tunnel: [w103 w139 w254 w283 w307 w336 w352 w375 w424 w475 w500 w509 w525] -> w68
      tunnel: w67 -> [w100 w137 w237 w281 w302 w322 w340 w369 w423 w472 w490 w507 w524]
      tunnel: [w94 w124 w237 w281 w302 w322 w340 w369 w423 w472 w490 w507 w524] -> w66
      tunnel: w65 -> [w92 w123 _ w280 w301 w321 w339 w362 w406 w471 w489 w506 w523]
      tunnel: [w92 w123 w228 w280 w301 w321 w339 w362 w406 w471 w489 w506 w523] -> w64
      event "Gamma", "Operator G Correction", "FrameCtl": Value Change {
        w113 = i8 0 ("[IN] Number of event")
        n52 = event-data() -> ()  [unwired: 1 in, 1 out]
        n53 = Decrement(x=w116) -> (x-1=w120:u32)
        n54 = property on="FrameCtl" class="DigNum (strict)"(error in=w115, "Maximum"=w120, "Minimum"=0.0 ("Data Entry Limits:Minimum")) -> ()  [unwired: 1 in, 2 out]
        n55 = call "Get_Preinitialized_Images-1.vi"("error IN"=w115, "[IN] Number of event"=w113, "[IN] Images Array"=w114) -> ("error OUT"=w108:errorcluster, "[OUT] Processed Image #1"=w112:T2, "[OUT] Source Image #2"=w107:T2)  [unwired: 1 in, 2 out]
        n56 = Number To Decimal String(number=w113) -> (decimal integer string=w110:string)  [unwired: 1 in]
        n57 = call "Refresh_Image_by_Copying_Fresh_One-1.vi"("[IN] Image Type"=w109, "[IN] Unique ID\n(# of Event)"=w110, "error IN"=w108, "Frame Number"="FrameCtl", "[IN] Preinitialized Image"=w107, "[IN] AVI Refnum"=w106) -> ("error OUT"=w101:errorcluster, "[OUT] Frame"=w102:T2)  [unwired: 1 in, 1 out]
        n58 = call "Refresh_Image_by_Copying_Fresh_One-1.vi"("[IN] Image Type"=w109, "[IN] Unique ID\n(# of Event)"=w110, "error IN"=w108, "Frame Number"="FrameCtl", "[IN] Preinitialized Image"=w112, "[IN] AVI Refnum"=w106) -> ("[OUT] Frame"=→"1st Movie (Comparison)":T2)  [unwired: 1 in, 2 out]
        n59 = call "Modify_Image_Histogram-3.vi"("[IN] Parameter"="Gamma", "[IN] Operator"="Operator G Correction", "1 - Origin\n2 - LoG"=u8 1 ("# channel"), "error IN"=w101, "[IN] Image Filtering Settings"=w100, "[IN] LoG Processed Image"=w102) -> ("error OUT"=w93:errorcluster, "[OUT] Image Filtering Settings"=w94:T12, "[OUT] Histogram Modified Image"=→"1st Movie":T2)  [unwired: 2 in, 1 out]
      }
      event "Gray or Binarized?", "FrameCtl2", "Sigma", "Index for thresholding", "Keep Nega-\ntive Values?", "Operator LoG", "Parameter LoG": Value Change {
        w138 = u32 0 items=["Grayscale", "Binary", "Gradient", "Rainbow", "Temperature", "User Defined"] ("Palette:Palette Type")
        w142 = u32 1 items=["Grayscale", "Binary", "Gradient", "Rainbow", "Temperature", "User Defined"] ("Palette:Palette Type")
        w148 = i8 1 ("[IN] Number of event")
        n60 = event-data() -> ()  [unwired: 1 in, 1 out]
        n61 = Decrement(x=w152) -> (x-1=w158:u32)
        n62 = property on="FrameCtl2" class="DigNum (strict)"(error in=w151, "Maximum"=w158, "Minimum"=0.0 ("Data Entry Limits:Minimum")) -> ()  [unwired: 1 in, 2 out]
        n63 = Number To Decimal String(number=w148) -> (decimal integer string=w126:string)  [unwired: 1 in]
        n64 = call "Get_Preinitialized_Images-1.vi"("error IN"=w151, "[IN] Number of event"=w148, "[IN] Images Array"=w150) -> ("error OUT"=w149:errorcluster, "[OUT] Processed Image #1"=w146:T2, "[OUT] Source Image #2"=w129:T2, "[OUT] Source Image #1"=w147:T2)  [unwired: 1 in, 1 out]
        n65 = Not(x="Gray or Binarized?") -> (.not. x?=w160:bool)
        n66 = case shown="False" w160 {
          tunnel: w149 -> [w201 w227]
          tunnel: [w196 w206] -> w132
          tunnel: [w200 w207] -> w133
          tunnel: "Sigma" -> [w174 w211]
          tunnel: "FrameCtl2" -> [w192 w221]
          tunnel: "Index for thresholding" -> [w187 _]
          tunnel: w154 -> [w185 w226]
          tunnel: [w182 w226] -> w153
          tunnel: w127 -> [w191 w220]
          tunnel: w125 -> [w181 w223]
          tunnel: w126 -> [w194 w225]
          tunnel: w147 -> [w193 w222]
          tunnel: w146 -> [w176 w210]
          tunnel: "Keep Nega-\ntive Values?" -> [w173 w213]
          tunnel: "Parameter LoG" -> [w162 w202]
          tunnel: "Operator LoG" -> [w163 w203]
          tunnel: w142 -> [w189 _]
          tunnel: w138 -> [_ w219]
          tunnel: w137 -> [w168 w208]
          tunnel: [w167 w204] -> w136
          frame False {
            n67 = property on="1st Movie Processed" class="ImageControl"(error in=w201, "Palette Type"=w189) -> (error out=w195:errorcluster)  [unwired: 1 in, 1 out]
            n68 = call "Refresh_Image_by_Copying_Fresh_One-1.vi"("[IN] Image Type"=w181, "[IN] Unique ID\n(# of Event)"=w194, "error IN"=w195, "Frame Number"=w192, "[IN] Preinitialized Image"=w193, "[IN] AVI Refnum"=w191) -> ("error OUT"=w178:errorcluster, "[OUT] Frame"=w180:T2)  [unwired: 1 in, 1 out]
            n69 = call "Modify_Image_Histogram-4.vi"("1 - Origin\n2 - LoG"=u8 1 ("# channel"), "error IN"=w178, "[IN] Image Filtering Settings"=w168, "[IN] LoG Processed Image"=w180) -> ("error OUT"=w175:errorcluster, "[OUT] Histogram Modified Image"=w177:T2)  [unwired: 5 in, 1 out]
            n70 = call "Localize_Particles-10.vi"("Keep Nega-\ntive Values?"=w173, "error IN"=w175, "[IN] Sigma"=w174, "[IN] Destination Image"=w176, "[IN] Frame"=w177) -> ("error OUT"=w169:errorcluster, "[OUT] LoG Processed Image"=w172:T2)  [unwired: 3 in, 1 out]
            n71 = call "Modify_Image_Histogram-3.vi"("[IN] Parameter"=w162, "[IN] Operator"=w163, "1 - Origin\n2 - LoG"=u8 2 ("1 - Origin\n2 - LoG"), "error IN"=w169, "[IN] Image Filtering Settings"=w168, "[IN] LoG Processed Image"=w172) -> ("error OUT"=w166:errorcluster, "[OUT] Image Filtering Settings"=w167:T12, "[OUT] Histogram"=w165:T15, "[OUT] Histogram Modified Image"=w164:T2)  [unwired: 2 in]
            n72 = call "Get_Initial_Value_For_Thresholding-1.vi"("[IN] Histogram Graph"=w165, "error IN"=w166) -> ("[OUT] Index of starting \npoint for thresholding"=w188:i32, "[OUT] Minimal index for \nthresholding (negative)"=w199:i32, "[OUT] Maximal index \nfor thresholding"=w198:i32, "error OUT"=w190:errorcluster)
            n73 = property on="Index for thresholding" class="DigNum (strict)"(error in=w190, "Maximum"=w198, "Minimum"=w199) -> (error out=w186:errorcluster)  [unwired: 1 in, 1 out]
            n74 = call "Get_Intensity_Value_For_Thresholding-2.vi"("[IN] Index for \nthresholding"=w187, "error IN"=w186, "[IN] Binarization Set\ntings (Both Channels)"=w185, "[IN] 1 or 2 channel"=u8 1, "[IN] Index of starting \npoint for thresholding"=w188) -> ("error OUT"=w183:errorcluster, "[OUT] Binarization Set\ntings (Both Channels)"=w182:cluster{"MinBin2":sgl, "MaxBin2":sgl}[], "[OUT] For Operator \nBinarization Values"=w184:cluster{"MinBin2":sgl, "MaxBin2":sgl})  [unwired: 1 in]
            n75 = call "IMAQ Threshold"("Replace Value"=sgl 9.0, "error in (no error)"=w183, "Range"=w184, "Image Src"=w164) -> ("error out"=w196:errorcluster, "Image Dst Out"=w200:T2)  [unwired: 6 in]
          }
          frame True {
            n76 = property on="1st Movie Processed" class="ImageControl"(error in=w227, "Palette Type"=w219) -> (error out=w224:errorcluster)  [unwired: 1 in, 1 out]
            n77 = call "Refresh_Image_by_Copying_Fresh_One-1.vi"("[IN] Image Type"=w223, "[IN] Unique ID\n(# of Event)"=w225, "error IN"=w224, "Frame Number"=w221, "[IN] Preinitialized Image"=w222, "[IN] AVI Refnum"=w220) -> ("error OUT"=w218:errorcluster, "[OUT] Frame"=w217:T2)  [unwired: 1 in, 1 out]
            n78 = call "Modify_Image_Histogram-4.vi"("1 - Origin\n2 - LoG"=u8 1 ("# channel"), "error IN"=w218, "[IN] Image Filtering Settings"=w208, "[IN] LoG Processed Image"=w217) -> ("error OUT"=w212:errorcluster, "[OUT] Histogram Modified Image"=w214:T2)  [unwired: 5 in, 1 out]
            n79 = call "Localize_Particles-10.vi"("Keep Nega-\ntive Values?"=w213, "error IN"=w212, "[IN] Sigma"=w211, "[IN] Destination Image"=w210, "[IN] Frame"=w214) -> ("error OUT"=w205:errorcluster, "[OUT] LoG Processed Image"=w209:T2)  [unwired: 3 in, 1 out]
            n80 = call "Modify_Image_Histogram-3.vi"("[IN] Parameter"=w202, "[IN] Operator"=w203, "1 - Origin\n2 - LoG"=u8 2 ("# channel"), "error IN"=w205, "[IN] Image Filtering Settings"=w208, "[IN] LoG Processed Image"=w209) -> ("error OUT"=w206:errorcluster, "[OUT] Image Filtering Settings"=w204:T12, "[OUT] Histogram Modified Image"=w207:T2)  [unwired: 2 in, 1 out]
          }
        }
        "1st Movie Processed" <- w133
        n81 = call "Refresh_Image_by_Copying_Fresh_One-1.vi"("[IN] Image Type"=w125, "[IN] Unique ID\n(# of Event)"=w126, "error IN"=w132, "Frame Number"="FrameCtl2", "[IN] Preinitialized Image"=w129, "[IN] AVI Refnum"=w127) -> ("error OUT"=w130:errorcluster, "[OUT] Frame"=→"1st Movie Original":T2)  [unwired: 1 in, 1 out]
        n82 = call "Modify_Image_Thresholding_Settings-2.vi"("[IN] Image Filtering Settings"=w136, "[IN] Index for thresholding"="Index for thresholding", "[IN] Sigma"="Sigma") -> ("[OUT] Image Filtering Settings"=w124:T12)  [unwired: 6 in]
      }
      event "Try my filters!", "Connectivity", "# Erosion", "Find ALL objects", "Save pics (ex)", "# of Frame": Value Change {
        n83 = event-data() -> ()  [unwired: 1 in, 1 out]
        n84 = Unbundle By Name(w229) -> ("Particle Fil Setups"=w234:T16)
        n85 = Decrement(x=w233) -> (x-1=w265:u32)
        n86 = call "Get_Values_Particle_Filter-1.vi"("Max  Diam"="Max  Diam", "Min  Diam"="Min  Diam") -> ("type of filters\nparticles search"=w251:T17)
        n87 = control-ref of="Detection Progress"() -> (w235:refnum<vi>)
        n88 = property on="# of Frame" class="DigNum (strict)"(error in=w244, "Maximum"=w265, "Minimum"=0.0 ("Data Entry Limits:Minimum")) -> (error out=w257:errorcluster)  [unwired: 1 in, 1 out]
        n89 = call "Merge_Particle_Filter_Setups-1.vi"("[IN] Particle Filter Setups"=w234, "type of filters\nparticles search"=w251, "Connectivity"="Connectivity", "# Erosion"="# Erosion") -> ("[OUT] Particle Filter Setups"=w250:T16)  [unwired: 3 in]
        n90 = property on="Keep Nega-\ntive Values?" class="Bool (strict)"(error in=w257) -> (error out=w236:errorcluster, "Value"=w248:bool)  [unwired: 1 in, 1 out]
        n91 = call "Merge_Localization_Settings_in_Cluster-1.vi"("[IN] Binarization Settings"=w247, "[IN] AVI Refnum"=w238, "[IN] Image Filtering Settings"=w237, "[IN] Image Type"=w246, "[IN] Keep Nega-\ntive Values?"=w248, "[IN] # Channel"=u8 1 ("# Channel"), "[IN] Particle Filter Setups"=w250) -> ("[OUT] Localization Settings"=w228:T8)  [unwired: 4 in]
        n92 = call "Visualize_Results_of_Filtering-1.vi"("[IN] Number of event"=i8 2, "error IN"=w244, "[IN] Localization Settings"=w228, "# Frame"="# of Frame", "[IN] Images Array"=w243) -> ("error OUT"=w239:errorcluster, "[OUT] LoG with Particles"=w240:T2, "[OUT] Binarized Image"=→"1st Filtering":T2)  [unwired: 4 in]
        "Results on 1st Movie" <- w240
        n93 = call "Localization_of_Objects-1.vi"("[IN] Detection Progress"=w235, "[IN] Number of Frames"=w233, "error IN"=w236, "[IN] Find ALL objects"="Find ALL objects", "[IN] Movie Related Values"=w229, "[IN] Localization Settings"=w228) -> ("error OUT"=w232:errorcluster, "[OUT] Movie Related Values"=w231:T11)  [unwired: 4 in]
        n94 = Merge Errors(w239, w232) -> (w258:errorcluster)
        n95 = case shown="True" "Save pics (ex)" {
          tunnel: w258 -> [w267 w269]
          tunnel: [w267 w270] -> w262
          tunnel: w240 -> [_ w268]
          frame False {
          }
          frame True {
            n96 = call "SavePics1.vi"("error IN"=w269, "default name"="Proces_Img2", "Image Dst IN"=w268) -> ("error out"=w270:errorcluster)  [unwired: 1 in]
          }
        }
      }
      event "Tracking Procedure": Value Change {
        n97 = event-data() -> ()  [unwired: 1 in, 1 out]
        n98 = control-ref of="Max angle"() -> (w295:refnum<vi>)
        n99 = control-ref of="Closing gaps"() -> (w297:refnum<vi>)
        n100 = control-ref of="Min TRK L"() -> (w294:refnum<vi>)
        n101 = control-ref of="dR min"() -> (w286:refnum<vi>)
        n102 = control-ref of="dR max"() -> (w285:refnum<vi>)
        n103 = control-ref of="% linearity"() -> (w296:refnum<vi>)
        n104 = call "Buttons_Limits(Tracking_Page)-1.vi"("[IN] dR max"=w285, "[IN] % linearity"=w296, "[IN] dR min"=w286, "[IN] Min TRK L"=w294, "error IN"=w299, "[IN] Number of Frames"=w298, "[IN] Max angle"=w295, "[IN] Closing gaps"=w297) -> ("error OUT"=w279:errorcluster)  [unwired: 3 in]
        n105 = control-ref of="Tracking progress"() -> (w287:refnum<vi>)
        n106 = Bundle("dR min"="dR min", "dR max"="dR max", "Closing gaps"="Closing gaps", "Min TRK L"="Min TRK L", "% linearity"="% linearity", "Max angle"="Max angle", "Tracking progress"=w287) -> (w276:T10)  [unwired: 1 in]
        n107 = call "Tracking_SubVI-4.vi"("[IN] Control Parameters"=w276, "error IN"=w279, "[IN] Before-After Tracks"=w278, "[IN] Movie Values"=w277) -> ("error OUT"=w273:errorcluster, "[OUT] Before-After Tracks"=w274:T13, "[OUT] Obtained Movie Values"=w275:T11, "[OUT] Number of \nRaw Displacements"=→"Raw #":i32)  [unwired: 4 in]
      }
      event "Filter Tracks": Value Change {
        n108 = event-data() -> ()  [unwired: 1 in, 1 out]
        n109 = call "Apply_Filters_to_Tracks-3.vi"("error IN"=w310, "[IN] Control Parameters"=w311, "[IN] Movie Values"=w312) -> ("error OUT"=w306:errorcluster, "[OUT] Filtered Tracks"=w307:T18, "[OUT] # Displ \nafter Filtration"=→"Saved #":i32, "[OUT] Filtered Movie Values"=w308:T11)  [unwired: 4 in, 1 out]
        n110 = control-ref of="Save pictures"() -> (w317:refnum<vi>)
        n111 = control-ref of="Delete Tracs"() -> (w316:refnum<vi>)
        n112 = control-ref of="Raw #"() -> (w320:refnum<vi>)
        n113 = control-ref of="Saved #"() -> (w319:refnum<vi>)
        n114 = control-ref of="Frame"() -> (w318:refnum<vi>)
        n115 = call "Disactivate_Frames_Until_Get_Tracking_Results-1.vi"("Delete Tracs Ref"=w316, "Save pictures Ref"=w317, "error IN"=w306, "Frame Ref"=w318, "Saved #  Ref"=w319, "Raw # Ref"=w320) -> ()  [unwired: 6 in]
        n116 = call "Calculation_Tracks_Statistics-4.vi"("error IN"=w306, "[IN] Tracks Statistics"=w304, "[IN] Filtered Tracks"=w307, "[IN] Movie Values"=w308) -> ("error OUT"=w305:errorcluster, "[OUT] Tracks Statistics"=w303:T14)  [unwired: 6 in]
      }
      event "dR min", "dR max", "Min TRK L", "Max angle", "% linearity": Value Change {
        n117 = event-data() -> ()  [unwired: 1 in, 1 out]
        n118 = property on="dR min" class="DigNum (strict)"(error in=w326) -> ("Value"=w337:dbl)  [unwired: 1 in, 2 out]
        n119 = property on="dR max" class="DigNum (strict)"(error in=w326) -> ("Value"=w331:dbl)  [unwired: 1 in, 2 out]
        n120 = property on="Max angle" class="DigNum (strict)"(error in=w326) -> ("Value"=w325:dbl)  [unwired: 1 in, 2 out]
        n121 = property on="% linearity" class="DigNum (strict)"(error in=w326) -> ("Value"=w327:i32)  [unwired: 1 in, 2 out]
        n122 = property on="Min TRK L" class="DigNum (strict)"(error in=w326) -> ("Value"=w328:i32)  [unwired: 1 in, 2 out]
        n123 = Unbundle(w338) -> ("Closing gaps"=w330:i32, "Tracking progress"=w329:refnum<vi>)  [unwired: 5 out]
        n124 = Bundle(cluster=w338, "dR min"=w337, "dR max"=w331, "Closing gaps"=w330, "Min TRK L"=w328, "% linearity"=w327, "Max angle"=w325, "Tracking progress"=w329) -> (w323:T10)
      }
      event "Show Distributions", "Bins": Value Change {
        n125 = event-data() -> ()  [unwired: 1 in, 1 out]
        n126 = call "Calculation_Statistic_Values-2.vi"("Intervals"="Bins", "[IN] Tracks Statistics"=w351) -> ("[OUT] Representation"=w349:T19)  [unwired: 3 in]
        n127 = Unbundle(w349) -> ("All Instant Vel-s"=→"All Instant Vels":T4, "mean"=→"mean Instant Vel":dbl, "standard deviation"=→"StD Instant":dbl, "All Path Vel-s"=→"All Path Vels":T4, "mean"=→"mean Path Vel":dbl, "standard deviation"=→"StD Path":dbl, "Mean Instan Vel-s"=→"Mean Instant Velocities for Each Track":T4, "Duration of tracks"=→"Duration of Tracks":T4)  [unwired: 4 out]
      }
      event "Frame", "Delete Tracs", "Save pictures": Value Change {
        w366 = i8 3 ("[IN] Number of event")
        n128 = event-data() -> ()  [unwired: 1 in, 1 out]
        n129 = Decrement(x=w383) -> (x-1=w387:u32)
        n130 = property on="Frame" class="DigNum (strict)"(error in=w368, "Maximum"=w387, "Minimum"=0.0 ("Data Entry Limits:Minimum")) -> ()  [unwired: 1 in, 2 out]
        n131 = Unbundle By Name(w389) -> ("Tracks, Coordinates"=w385:T20)
        n132 = call "Visualize_Results_of_Filtering-1.vi"("[IN] Number of event"=w366, "error IN"=w368, "[IN] Localization Settings"=w362, "# Frame"="Frame", "[IN] Images Array"=w361) -> ("error OUT"=w364:errorcluster, "[OUT] LoG with Particles"=w367:T2)  [unwired: 4 in, 1 out]
        n133 = Increment(x=w366) -> (x+1=w365:i8)
        n134 = Unbundle By Name(w385) -> ("(X,Y,dX,dY) NN filtered"=w371:dbl[][], "(X,Y,dX,dY) TH filtered"=w381:dbl[][])
        n135 = call "Visualize_Results_of_Filtering-1.vi"("[IN] Number of event"=w365, "error IN"=w364, "[IN] Localization Settings"=w362, "# Frame"="Frame", "[IN] Images Array"=w361) -> ("error OUT"=w360:errorcluster, "[OUT] LoG with Particles"=w359:T2)  [unwired: 4 in, 1 out]
        n136 = call "Paint_Tracks_on_Frame-1.vi"("Delete \nOverlay?"="Delete Tracs", "[IN] Number of event"=i8 24, "[IN] Images Array"=w361, "error IN"=w360, "# Frame"="Frame", "[IN] #1 Array (X,Y,...)"=w371, "[IN] #1 Processed Image"=w367) -> ("error OUT"=w373:errorcluster, "[OUT] #1 Overlayed Image"=w374:T2)  [unwired: 2 in]
        "1st Filtering (NN)" <- w374
        n137 = call "Paint_Tracks_on_Frame-1.vi"("Delete \nOverlay?"="Delete Tracs", "[IN] Number of event"=i8 21, "[IN] Images Array"=w361, "error IN"=w373, "# Frame"="Frame", "[IN] #1 Array (X,Y,...)"=w381, "[IN] #1 Processed Image"=w359) -> ("error OUT"=w378:errorcluster, "[OUT] #1 Overlayed Image"=w379:T2)  [unwired: 2 in]
        "1st Filtered" <- w379
        n138 = case shown="True" "Save pictures" {
          tunnel: w379 -> [_ w399]
          tunnel: w374 -> [_ w396]
          tunnel: w378 -> [w392 w398]
          tunnel: [w392 w393] -> w390
          frame False {
          }
          frame True {
            n139 = call "SavePics1.vi"("error IN"=w398, "default name"="Track_Img1", "Image Dst IN"=w399) -> ("error out"=w394:errorcluster)  [unwired: 1 in]
            n140 = call "SavePics1.vi"("error IN"=w394, "default name"="Track_Img2", "Image Dst IN"=w396) -> ("error out"=w393:errorcluster)  [unwired: 1 in]
          }
        }
      }
      event "Testing Frame", "Save pics below", "Tracks group", "Save videos \nbelow as *avi": Value Change {
        w418 = i8 5 ("[IN] Number of event")
        n141 = event-data() -> ()  [unwired: 1 in, 1 out]
        n142 = Unbundle(w428) -> ("Before Grouped Tracks"=w419:T21, "After Grouped Tracks"=w414:T21, "Current\nGroup"=w441:i32)
        n143 = Array Size(array=w419) -> (size(s)=w437:i32)
        n144 = call "Get_Info_Before-After_Tracks-1.vi"("[IN] After Tracks"=w414, "[IN] Tracks group"="Tracks group", "[IN] Before Tracks"=w419) -> ("[OUT] Maximal Frame\n(finish point all tracks)"=w435:i32, "[OUT] Min Start Pos"=w434:i32)
        n145 = Decrement(x=w437) -> (x-1=w436:i32)
        n146 = property on="Tracks group" class="DigNum (strict)"(error in=w422, "Maximum"=w436, "Minimum"=0.0 ("Data Entry Limits:Minimum")) -> (error out=w442:errorcluster)  [unwired: 1 in, 1 out]
        n147 = property on="Keep Nega-\ntive Values?" class="Bool (strict)" props=["Value"](error in=w422) -> ()  [unwired: 1 in, 3 out]
        n148 = property on="Testing \nFrame" class="DigNum (strict)"(error in=w442, "Maximum"=w435, "Minimum"=w434) -> (error out=w440:errorcluster)  [unwired: 1 in, 1 out]
        n149 = To Unsigned Long Integer(number=w434) -> (unsigned 32bit integer=w433:u32)
        n150 = property on="Tracks \ngroup" class="DigNum (strict)"(error in=w440) -> (error out=w438:errorcluster, "Value"=w427:i32)  [unwired: 1 in, 1 out]
        n151 = in-place {
          in-place-border: w427 -> [w447]
          n152 = in-place-cluster #1(w428) -> ()  [unwired: 1 out]
          n153 = in-place-cluster #1("Current\nGroup"=w447) -> (w426:T13)
        }
        n154 = Equal?(x=w427, y=w441) -> (x = y?=w432:bool)
        n155 = case shown="True" w432 {
          tunnel: w438 -> [w450 w452]
          tunnel: w433 -> [w448 _]
          tunnel: [w449 w452] -> w421
          tunnel: [w448 w451] -> w416
          tunnel: "Testing Frame" -> [_ w451]
          frame False {
            n156 = property on="Testing \nFrame" class="DigNum (strict)"(error in=w450, "Value"=w448) -> (error out=w449:errorcluster)  [unwired: 1 in, 1 out]
          }
          frame True {
          }
        }
        n157 = call "Merge_Grouped_Tracks_Values-1.vi"("[IN] Testing Frame"=w416, "[IN] Tracks group"="Tracks group", "[IN] Grouped Tracks"=w419) -> ("[OUT] Grouped Tracks Values"=w411:T22)  [unwired: 2 in]
        n158 = call "Merge_Grouped_Tracks_Values-1.vi"("[IN] Testing Frame"=w416, "[IN] Tracks group"="Tracks group", "[IN] Grouped Tracks"=w414) -> ("[OUT] Grouped Tracks Values"=w405:T22)  [unwired: 2 in]
        n159 = call "Paint_Tracks_Before-After-4.vi"("[IN] Number of event"=w418, "[IN] Localization Settings"=w406, "[IN] Images Array"=w403, "error IN"=w421, "[IN] Grouped Tracks Values"=w411) -> ("error OUT"=w417:errorcluster, "[OUT] Image with\nDisplacements"=w420:T2)  [unwired: 5 in]
        "Connected and Grouped Tracks" <- w420
        n160 = Increment(x=w418) -> (x+1=w409:i8)
        n161 = call "Paint_Tracks_Before-After-4.vi"("[IN] Number of event"=w409, "[IN] Localization Settings"=w406, "[IN] Images Array"=w403, "error IN"=w417, "[IN] Grouped Tracks Values"=w405) -> ("error OUT"=w412:errorcluster, "[OUT] Image with\nDisplacements"=w413:T2)  [unwired: 5 in]
        "After Resolving Correspondence Problem" <- w413
        n162 = Increment(x=w409) -> (x+1=w402:i8)
        n163 = call "Save_Before-After_Tracks-4.vi"("Save movies?"="Save videos \nbelow as *avi", "[IN] Number of event"=w402, "[IN] Localization Settings"=w406, "[IN] Images Array"=w403, "error IN"=w412, "[IN] FPS"="FPS Gr", "default name"="Tracks_Before_Filt", "[IN] Grouped Tracks Values"=w411) -> ("error OUT"=w408:errorcluster)  [unwired: 3 in]
        n164 = case shown="True" "Save pics below" {
          tunnel: w420 -> [_ w456]
          tunnel: w412 -> [w453 w458]
          tunnel: [w453 w457] -> w439
          tunnel: w413 -> [_ w455]
          frame False {
          }
          frame True {
            n165 = Two Button Dialog(message="1 or 2?", 1:"After" ("F button name (\"Cancel\")"), 2:"Before" ("T button name (\"OK\")")) -> (T button?=w460:bool)
            n166 = case shown="True" w460 {
              tunnel: "Trck_ImgN" ("default name") -> [w465 w470]
              tunnel: w458 -> [w466 w469]
              tunnel: [w463 w468] -> w457
              tunnel: w456 -> [_ w467]
              tunnel: w455 -> [w464 _]
              frame False {
                n167 = call "SavePics1.vi"("error IN"=w466, "default name"=w465, "Image Dst IN"=w464) -> ("error out"=w463:errorcluster)  [unwired: 1 in]
              }
              frame True {
                n168 = call "SavePics1.vi"("error IN"=w469, "default name"=w470, "Image Dst IN"=w467) -> ("error out"=w468:errorcluster)  [unwired: 1 in]
              }
            }
          }
        }
        n169 = Increment(x=w402) -> (x+1=w401:i8)
        n170 = call "Save_Before-After_Tracks-4.vi"("Save movies?"="Save videos \nbelow as *avi", "[IN] Number of event"=w401, "[IN] Localization Settings"=w406, "[IN] Images Array"=w403, "error IN"=w408, "[IN] FPS"="FPS Gr", "default name"="Tracks_After_Filt", "[IN] Grouped Tracks Values"=w405) -> ()  [unwired: 3 in, 1 out]
      }
      event "Save movies": Value Change {
        n171 = event-data() -> ()  [unwired: 1 in, 1 out]
        n172 = Unbundle By Name(w487) -> ("Tracks, Coordinates"=w474:T20)
        n173 = Unbundle By Name(w474) -> ("(X,Y,dX,dY) TH filtered"=w483:dbl[][])
        n174 = call "Save_Tracking_Results_Movie-2.vi"("Save movies"="Save movies", "FPS"="FPS", "# codec"=4, "error IN"=w484, "AVI Refnum"=w481, "default name"="Processed_Movie1", "(X,Y,dX,dY)"=w483) -> ("error out"=w478:errorcluster)  [unwired: 4 in]
      }
      event "Save All Instant Vels", "Save Path Velocities", "Save Mean Velocities", "Save Duration of Tracks", "Save Tracks in Columns (x,y,dx,dy)": Value Change {
        n175 = event-data() -> ()  [unwired: 1 in, 1 out]
        n176 = call "Save_Various_Calculated_Vals_1.vi"("[IN] Save Tracks in Columns"="Save Tracks in Columns (x,y,dx,dy)", "[IN] Save Mean Vels for Tracks"="Save Mean Velocities", "[IN] Save Track Durations"="Save Duration of Tracks", "[IN] Save All Path Velocities"="Save Path Velocities", "error IN"=w496, "[IN] Statistics"=w498, "[IN] Save All Instant Velocities"="Save All Instant Vels", "[IN] File Path with Movie"=w495) -> ("error OUT"=w497:errorcluster)  [unwired: 3 in]
      }
      event "STOP Program": Value Change {
        n177 = event-data() -> ()  [unwired: 1 in, 1 out]
        n178 = Index Array(array=w517, index=0) -> (element=w513:T2)
        n179 = call "IMAQ AVI2 Close"("error in (no error)"=w515, "AVI Refnum"=w516) -> ("error out"=w512:errorcluster)  [unwired: 9 in]
        n180 = Request Deallocation("STOP Program") -> ()
        n181 = call "IMAQ Dispose"("All Images? (No)"=TRUE, "Image"=w513, "error in (no error)"=w512) -> ("error out"=w511:errorcluster)  [unwired: 3 in]
      }
      event Timeout {
        n182 = event-data() -> ()  [unwired: 1 in, 1 out]
      }
    }
    "error out" <- w80
    n183 = Unbundle(w80) -> ("code"=w87:i32, "source"=w86:string)  [unwired: 1 out]
    n184 = call <vilib>:"Simple Error Handler.vi"("error code (no error:0)"=w87, "error source (\" \")"=w86, "error in (no error)"=w80) -> ()  [unwired: 2 in, 5 out]
  }
